vi "Parse Loaded Profile (uSMC).vi"(2 "replace(false)/insert(true)":bool, 3 "SMindex":i32, 4 "Version":string, 5 "data string":string) -> ()   [LabVIEW 2010, in "SignalWriterMH110203USBStepperMotor.lvclass"]
uses:
  SignalWriterMH110203USBStepperMotor.lvclass
  Get State Control (uSMC).ctl
  Set Parameters (uSMC).ctl
  class_data.vi
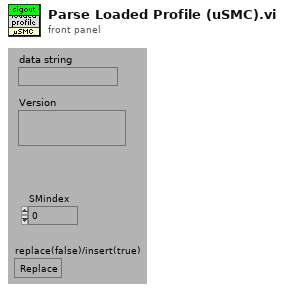
[diagram p1: front panel]
types:
  T1 = typedef "SignalWriterMH110203USBStepperMotor.lvclass/Get State Control (uSMC).ctl" = cluster{"Current Posistion":dbl, "CW/CCW":bool, "Speed":u16, "Temperature":dbl, "Power":u16, "Limit Switch 1":bool, "Limit Switch 2":bool, "After Reset":bool, "Step":u8, "Backlash":bool, "RT Error":bool, "RT State":bool, "Sync In":bool, "Sync Out":bool, "Ext Disconnect":bool, "Usb Powered":bool, "Voltage":dbl, "Working":bool, "SM Position in Encoder Units":i32, "Encoder Current Position":i32}
  T2 = typedef "SignalWriterMH110203USBStepperMotor.lvclass/Set Parameters (uSMC).ctl" = cluster{"Acceleration Time":u8, "Deceleration Time":u8, "Reduce Current Timeout":u16, "Buttons Timeout 1":u16, "Buttons Timeout 2":u16, "Buttons Timeout 3":u16, "Buttons Timeout 4":u16, "Buttons Timeout Reset":u16, "Buttons Timeout DblClick":u16, "Reset Speed":u16, "Buttons Speed 1":u16, "Buttons Speed 2":u16, "Buttons Speed 3":u16, "Buttons Speed 4":u16, "Max Backlash":u16, "Start Pos":i32, "RTdelta":u16, "RTMinError":u16, "Maximum Temperature":u16, "Sync Duration":u8, "Backlash Speed":u16, "EncVSCP":u8, "Steps Per Revolution":i32, "Encoder Pulses Per Rev-on":i32}
  T3 = cluster{"Cur Pos Units":dbl, "Set Cur Pos units":dbl, "Lo Limit Units":dbl, "Hi Limit Units":dbl, "Cur Pos Ticks":i32, "Set Cur Pos ticks":i32, "Lo Limit Ticks":i32, "Hi Limit Ticks":i32, "Minimal Value":dbl, "Maximal Value":dbl}
  T4 = typedef "SignalWriterMH110203USBStepperMotor.lvclass/Mode Control (uSMC).ctl" = cluster{"Turn Buttons Off":bool, "Reduce Current":bool, "Power Off and Make a Whole Step":bool, "Emergency Power Off":bool, "Limit Switch 1 True State":bool, "Limit Switch 2 True State":bool, "Rotary Transducer TRUE State":bool, "Swap Limit Switches":bool, "Limit Switch 1 Operation Enabled":bool, "Limit Switch 2 Operation Enabled":bool, "Rotary Transducer Operation Enabled":bool, "Rotary Transducer Operation Select":bool, "Button 1 True State":bool, "Button 2 True State":bool, "Swap Buttons":bool, "Reset Rotary Transducer Check Positions":bool, "Output Syncronization Enabled":bool, "Reset Output Sync Count":bool, "Sync Operation":bool, "Sync Count":u32, "Power":bool, "Invert Sync Polarity":bool, "Use Encoder":bool, "Invert Encoder Direction":bool, "Reset Encoder To 0":bool, "Reset SM Enc Pos to Enc Pos":bool}
  T5 = typedef "SignalWriterMH110203USBStepperMotor.lvclass/GoTo Control (uSMC).ctl" = cluster{"Step motor ID":string, "SMname":string, "Backlash":u16, "wait for input sygnal to start":bool, "use slow start/stop":bool, "units name":string, "Maximum speed":dbl, "speed":dbl, "step":u8, "point 1 ticks":i32, "point 2 ticks":i32, "point 1 units":dbl, "point 2 units":dbl, "Limit Switch standoff":dbl, "Zero Value":dbl, "Destination Position":dbl, "force backlash":bool, "power off when stop":bool, "POff delay":dbl, "positioner name":string, "R, Ohm":dbl, "I, mA":dbl, "Positioner's Type":u16, "Reset Direction":bool, "Manufacturer":string, "Model":string, "Scheme":string, "FirmwareVer":string}
  T6 = cluster{"Step motor ID":string, "SMname":string, "Loft":u16, "wait for input sygnal to start":bool, "use slow start/stop":bool, "units name":string, "Maximum speed":dbl, "speed":dbl, "step":u8, "point 1 ticks":i32, "point 2 ticks":i32, "point 1 units":dbl, "point 2 units":dbl, "Trailer 1 standoff":dbl, "Zero Value":dbl, "Destination Position":dbl, "force loft":bool, "power off when stop":bool, "POff delay":dbl, "positioner name":string, "R, Ohm":dbl, "I, mA":dbl, "Positioner's Type":u16, "Reset Direction":bool, "Manufacturer":string, "Model":string, "Scheme":string}
  T7 = cluster{"cur pos units":dbl, "set cur pos units value":dbl, "lo limit units":dbl, "hi limit units":dbl, "cur pos ticks":i32, "set cur pos ticks value":i32, "lo limit ticks":i32, "hi limit ticks":i32, "Minimal Value":dbl, "Maximal Value":dbl}
  T8 = cluster{"Step motor ID":string, "SMname":string, "Loft":u16, "wait for input sygnal to start":bool, "use slow start/stop":bool, "units name":string, "Maximum speed":dbl, "speed":dbl, "step":u8, "point 1 ticks":i32, "point 2 ticks":i32, "point 1 units":dbl, "point 2 units":dbl, "Trailer 1 standoff":dbl, "Zero Value":dbl, "Destination Position":dbl, "force loft":bool, "power off when stop":bool, "POff delay":dbl, "positioner name":string, "R, Ohm":dbl, "I, mA":dbl, "Positioner's Type":u16, "Reset Direction":bool, "Manufacturer":string, "Model":string, "Scheme":string, "FirmwareVer":string}
  T9 = cluster{"Turn Buttons Off":bool, "Reduce Current":bool, "Power Off and Make a Whole Step":bool, "Emergency Power Off":bool, "Trailer 1 True State":bool, "Trailer 2 True State":bool, "Rotary Transducer TRUE State":bool, "Swap Trailers":bool, "Trailer 1 Operation Enabled":bool, "Trailer 2 Operation Enabled":bool, "Rotary Transducer Operation Enabled":bool, "Rotary Transducer Operation Select":bool, "Button 1 True State":bool, "Button 2 True State":bool, "Swap Buttons":bool, "Reset Rotary Transducer Check Positions":bool, "Output Syncronization Enabled":bool, "Reset Output Sync Count":bool, "Sync Operation":bool, "Sync Count":u32, "Power":bool, "Invert Sync Polarity":bool, "Use Encoder":bool, "Invert Encoder Direction":bool, "Reset Encoder To 0":bool, "Reset SM Enc Pos to Enc Pos":bool}
  T10 = cluster{"Step motor ID":string, "SMname":string, "Loft":u16, "wait for input sygnal to start":bool, "use slow start/stop":bool, "units name":string, "Maximum speed":dbl, "speed":dbl, "step":u8, "point 1 ticks":i32, "point 2 ticks":i32, "point 1 units":dbl, "point 2 units":dbl, "Trailer 1 standoff":dbl, "Trailer 2 standoff":dbl, "Destination Position":dbl, "force loft":bool, "power off when stop":bool, "POff delay":dbl}
  T11 = cluster{"cur pos units":dbl, "set cur pos units value":dbl, "lo limit units":dbl, "hi limit units":dbl, "cur pos ticks":i32, "set cur pos ticks value":i32, "lo limit ticks":i32, "hi limit ticks":i32}
  T12 = cluster{"Delay 1":u8, "Delay 2":u8, "RefINTimeout":u16, "BTIMEOUT 1":u16, "BTIMEOUT 2":u16, "BTIMEOUT 3":u16, "BTIMEOUT 4":u16, "BTIMEOUT R":u16, "BTIMEOUT D":u16, "Min period":u16, "BTO1P":u16, "BTO2P":u16, "BTO3P":u16, "BTO4P":u16, "Max Loft":u16, "Start Pos":i32, "RTDelta":u16, "RTMinError":u16, "Maximum temperature":u16, "sync duration":u8, "LoftPeriod":u16}
  T13 = cluster{"buttons off":bool, "RefIin current":bool, "power off and make a whole step":bool, "emergency power off":bool, "trailer 1 true state":bool, "trailer 2 true state":bool, "Rotary Transducer TRUE state":bool, "trailers swap":bool, "trailer 1 operation enabled":bool, "trailer 2 operation enabled":bool, "Rotary Transducer Operation enabled":bool, "Rotary Transducer Operation select":bool, "Button 1 TRUE state":bool, "Button 2 TRUE state":bool, "Buttons are Swapped":bool, "Reset Rotary Transducer Check Positions":bool, "Output Syncronization Enabled":bool, "reset output sync count":bool, "Sync operation true-one time, false - many times":bool, "Sync count":u32, "power state":bool}
  T14 = cluster{"SetMode defalults":cluster{"buttons off":bool, "RefIin current":bool, "power off and make a whole step":bool, "emergency power off":bool, "trailer 1 true state":bool, "trailer 2 true state":bool, "Rotary Transducer TRUE state":bool, "trailers swap":bool, "trailer 1 operation enabled":bool, "trailer 2 operation enabled":bool, "Rotary Transducer Operation enabled":bool, "Rotary Transducer Operation select":bool, "Button 1 TRUE state":bool, "Button 2 TRUE state":bool, "Buttons are Swapped":bool, "Reset Rotary Transducer Check Positions":bool, "Output Syncronization Enabled":bool, "reset output sync count":bool, "Sync operation true-one time, false - many times":bool, "Sync count":u32, "power state":bool}, "SetParams Defalut":cluster{"Delay 1":u8, "Delay 2":u8, "RefINTimeout":u16, "BTIMEOUT 1":u16, "BTIMEOUT 2":u16, "BTIMEOUT 3":u16, "BTIMEOUT 4":u16, "BTIMEOUT R":u16, "BTIMEOUT D":u16, "Min period":u16, "BTO1P":u16, "BTO2P":u16, "BTO3P":u16, "BTO4P":u16, "Max Loft":u16, "Start Pos":i32, "RTDelta":u16, "RTMinError":u16, "Maximum temperature":u16, "sync duration":u8, "LoftPeriod":u16}, "Position Default":cluster{"cur pos units":dbl, "set cur pos units value":dbl, "lo limit units":dbl, "hi limit units":dbl, "cur pos ticks":i32, "set cur pos ticks value":i32, "lo limit ticks":i32, "hi limit ticks":i32}, "GoToPlus default":cluster{"Step motor ID":string, "SMname":string, "Loft":u16, "wait for input sygnal to start":bool, "use slow start/stop":bool, "units name":string, "Maximum speed":dbl, "speed":dbl, "step":u8, "point 1 ticks":i32, "point 2 ticks":i32, "point 1 units":dbl, "point 2 units":dbl, "Trailer 1 standoff":dbl, "Trailer 2 standoff":dbl, "Destination Position":dbl, "force loft":bool, "power off when stop":bool, "POff delay":dbl}}
  T15 = cluster{"Step motor ID":string, "SMname":string, "Loft":u16, "wait for input sygnal to start":bool, "use slow start/stop":bool, "units name":string, "Maximum speed":dbl, "speed":dbl, "step":u8, "point 1 ticks":i32, "point 2 ticks":i32, "point 1 units":dbl, "point 2 units":dbl, "Trailer 1 standoff":dbl, "Trailer 2 standoff":dbl, "Destination Position":dbl, "force loft":bool, "power off when stop":bool, "POff delay":dbl, "positioner name":string}
  T16 = cluster{"SetMode defalults":cluster{"buttons off":bool, "RefIin current":bool, "power off and make a whole step":bool, "emergency power off":bool, "trailer 1 true state":bool, "trailer 2 true state":bool, "Rotary Transducer TRUE state":bool, "trailers swap":bool, "trailer 1 operation enabled":bool, "trailer 2 operation enabled":bool, "Rotary Transducer Operation enabled":bool, "Rotary Transducer Operation select":bool, "Button 1 TRUE state":bool, "Button 2 TRUE state":bool, "Buttons are Swapped":bool, "Reset Rotary Transducer Check Positions":bool, "Output Syncronization Enabled":bool, "reset output sync count":bool, "Sync operation true-one time, false - many times":bool, "Sync count":u32, "power state":bool}, "SetParams Defalut":cluster{"Delay 1":u8, "Delay 2":u8, "RefINTimeout":u16, "BTIMEOUT 1":u16, "BTIMEOUT 2":u16, "BTIMEOUT 3":u16, "BTIMEOUT 4":u16, "BTIMEOUT R":u16, "BTIMEOUT D":u16, "Min period":u16, "BTO1P":u16, "BTO2P":u16, "BTO3P":u16, "BTO4P":u16, "Max Loft":u16, "Start Pos":i32, "RTDelta":u16, "RTMinError":u16, "Maximum temperature":u16, "sync duration":u8, "LoftPeriod":u16}, "Position Default":cluster{"cur pos units":dbl, "set cur pos units value":dbl, "lo limit units":dbl, "hi limit units":dbl, "cur pos ticks":i32, "set cur pos ticks value":i32, "lo limit ticks":i32, "hi limit ticks":i32}, "GoToPlus default":cluster{"Step motor ID":string, "SMname":string, "Loft":u16, "wait for input sygnal to start":bool, "use slow start/stop":bool, "units name":string, "Maximum speed":dbl, "speed":dbl, "step":u8, "point 1 ticks":i32, "point 2 ticks":i32, "point 1 units":dbl, "point 2 units":dbl, "Trailer 1 standoff":dbl, "Trailer 2 standoff":dbl, "Destination Position":dbl, "force loft":bool, "power off when stop":bool, "POff delay":dbl, "positioner name":string}}
  T17 = cluster{"SetMode defalults":cluster{"buttons off":bool, "RefIin current":bool, "power off and make a whole step":bool, "emergency power off":bool, "trailer 1 true state":bool, "trailer 2 true state":bool, "Rotary Transducer TRUE state":bool, "trailers swap":bool, "trailer 1 operation enabled":bool, "trailer 2 operation enabled":bool, "Rotary Transducer Operation enabled":bool, "Rotary Transducer Operation select":bool, "Button 1 TRUE state":bool, "Button 2 TRUE state":bool, "Buttons are Swapped":bool, "Reset Rotary Transducer Check Positions":bool, "Output Syncronization Enabled":bool, "reset output sync count":bool, "Sync operation true-one time, false - many times":bool, "Sync count":u32, "power state":bool}, "SetParams Defalut":cluster{"Delay 1":u8, "Delay 2":u8, "RefINTimeout":u16, "BTIMEOUT 1":u16, "BTIMEOUT 2":u16, "BTIMEOUT 3":u16, "BTIMEOUT 4":u16, "BTIMEOUT R":u16, "BTIMEOUT D":u16, "Min period":u16, "BTO1P":u16, "BTO2P":u16, "BTO3P":u16, "BTO4P":u16, "Max Loft":u16, "Start Pos":i32, "RTDelta":u16, "RTMinError":u16, "Maximum temperature":u16, "sync duration":u8, "LoftPeriod":u16}, "Position Default":cluster{"cur pos units":dbl, "set cur pos units value":dbl, "lo limit units":dbl, "hi limit units":dbl, "cur pos ticks":i32, "set cur pos ticks value":i32, "lo limit ticks":i32, "hi limit ticks":i32, "Minimal Value":dbl, "Maximal Value":dbl}, "GoToPlus default":cluster{"Step motor ID":string, "SMname":string, "Loft":u16, "wait for input sygnal to start":bool, "use slow start/stop":bool, "units name":string, "Maximum speed":dbl, "speed":dbl, "step":u8, "point 1 ticks":i32, "point 2 ticks":i32, "point 1 units":dbl, "point 2 units":dbl, "Trailer 1 standoff":dbl, "Zero Value":dbl, "Destination Position":dbl, "force loft":bool, "power off when stop":bool, "POff delay":dbl, "positioner name":string, "R, Ohm":dbl, "I, mA":dbl, "Positioner's Type":u16, "Reset Direction":bool, "Manufacturer":string, "Model":string, "Scheme":string}}
  T18 = cluster{"SetMode defalults":cluster{"buttons off":bool, "RefIin current":bool, "power off and make a whole step":bool, "emergency power off":bool, "trailer 1 true state":bool, "trailer 2 true state":bool, "Rotary Transducer TRUE state":bool, "trailers swap":bool, "trailer 1 operation enabled":bool, "trailer 2 operation enabled":bool, "Rotary Transducer Operation enabled":bool, "Rotary Transducer Operation select":bool, "Button 1 TRUE state":bool, "Button 2 TRUE state":bool, "Buttons are Swapped":bool, "Reset Rotary Transducer Check Positions":bool, "Output Syncronization Enabled":bool, "reset output sync count":bool, "Sync operation true-one time, false - many times":bool, "Sync count":u32, "power state":bool}, "SetParams Defalut":cluster{"Delay 1":u8, "Delay 2":u8, "RefINTimeout":u16, "BTIMEOUT 1":u16, "BTIMEOUT 2":u16, "BTIMEOUT 3":u16, "BTIMEOUT 4":u16, "BTIMEOUT R":u16, "BTIMEOUT D":u16, "Min period":u16, "BTO1P":u16, "BTO2P":u16, "BTO3P":u16, "BTO4P":u16, "Max Loft":u16, "Start Pos":i32, "RTDelta":u16, "RTMinError":u16, "Maximum temperature":u16, "sync duration":u8, "LoftPeriod":u16}, "Position Default":cluster{"cur pos units":dbl, "set cur pos units value":dbl, "lo limit units":dbl, "hi limit units":dbl, "cur pos ticks":i32, "set cur pos ticks value":i32, "lo limit ticks":i32, "hi limit ticks":i32, "Minimal Value":dbl, "Maximal Value":dbl}, "GoToPlus default":cluster{"Step motor ID":string, "SMname":string, "Loft":u16, "wait for input sygnal to start":bool, "use slow start/stop":bool, "units name":string, "Maximum speed":dbl, "speed":dbl, "step":u8, "point 1 ticks":i32, "point 2 ticks":i32, "point 1 units":dbl, "point 2 units":dbl, "Trailer 1 standoff":dbl, "Zero Value":dbl, "Destination Position":dbl, "force loft":bool, "power off when stop":bool, "POff delay":dbl, "positioner name":string, "R, Ohm":dbl, "I, mA":dbl, "Positioner's Type":u16, "Reset Direction":bool, "Manufacturer":string, "Model":string, "Scheme":string, "FirmwareVer":string}}
  T19 = cluster{"buttons off":bool, "RefIin current":bool, "power off and make a whole step":bool, "emergency power off":bool, "trailer 1 true state":bool, "trailer 2 true state":bool, "Rotary Transducer TRUE state":bool, "trailers swap":bool, "trailer 1 operation enabled":bool, "trailer 2 operation enabled":bool, "Rotary Transducer Operation enabled":bool, "Rotary Transducer Operation select":bool, "Button 1 TRUE state":bool, "Button 2 TRUE state":bool, "Buttons are Swapped":bool, "Reset Rotary Transducer Check Positions":bool, "Output Syncronization Enabled":bool, "reset output sync count":bool, "Sync operation true-one time, false - many times":bool, "Sync count":u32, "power state":bool, "Const TTL output":bool}
  T20 = cluster{"SetMode defalults":cluster{"buttons off":bool, "RefIin current":bool, "power off and make a whole step":bool, "emergency power off":bool, "trailer 1 true state":bool, "trailer 2 true state":bool, "Rotary Transducer TRUE state":bool, "trailers swap":bool, "trailer 1 operation enabled":bool, "trailer 2 operation enabled":bool, "Rotary Transducer Operation enabled":bool, "Rotary Transducer Operation select":bool, "Button 1 TRUE state":bool, "Button 2 TRUE state":bool, "Buttons are Swapped":bool, "Reset Rotary Transducer Check Positions":bool, "Output Syncronization Enabled":bool, "reset output sync count":bool, "Sync operation true-one time, false - many times":bool, "Sync count":u32, "power state":bool, "Const TTL output":bool}, "SetParams Defalut":cluster{"Delay 1":u8, "Delay 2":u8, "RefINTimeout":u16, "BTIMEOUT 1":u16, "BTIMEOUT 2":u16, "BTIMEOUT 3":u16, "BTIMEOUT 4":u16, "BTIMEOUT R":u16, "BTIMEOUT D":u16, "Min period":u16, "BTO1P":u16, "BTO2P":u16, "BTO3P":u16, "BTO4P":u16, "Max Loft":u16, "Start Pos":i32, "RTDelta":u16, "RTMinError":u16, "Maximum temperature":u16, "sync duration":u8, "LoftPeriod":u16}, "Position Default":cluster{"cur pos units":dbl, "set cur pos units value":dbl, "lo limit units":dbl, "hi limit units":dbl, "cur pos ticks":i32, "set cur pos ticks value":i32, "lo limit ticks":i32, "hi limit ticks":i32, "Minimal Value":dbl, "Maximal Value":dbl}, "GoToPlus default":cluster{"Step motor ID":string, "SMname":string, "Loft":u16, "wait for input sygnal to start":bool, "use slow start/stop":bool, "units name":string, "Maximum speed":dbl, "speed":dbl, "step":u8, "point 1 ticks":i32, "point 2 ticks":i32, "point 1 units":dbl, "point 2 units":dbl, "Trailer 1 standoff":dbl, "Zero Value":dbl, "Destination Position":dbl, "force loft":bool, "power off when stop":bool, "POff delay":dbl, "positioner name":string, "R, Ohm":dbl, "I, mA":dbl, "Positioner's Type":u16, "Reset Direction":bool, "Manufacturer":string, "Model":string, "Scheme":string, "FirmwareVer":string}}
  T21 = cluster{"Mode Defalults":cluster{"Turn Buttons Off":bool, "Reduce Current":bool, "Power Off and Make a Whole Step":bool, "Emergency Power Off":bool, "Trailer 1 True State":bool, "Trailer 2 True State":bool, "Rotary Transducer TRUE State":bool, "Swap Trailers":bool, "Trailer 1 Operation Enabled":bool, "Trailer 2 Operation Enabled":bool, "Rotary Transducer Operation Enabled":bool, "Rotary Transducer Operation Select":bool, "Button 1 True State":bool, "Button 2 True State":bool, "Swap Buttons":bool, "Reset Rotary Transducer Check Positions":bool, "Output Syncronization Enabled":bool, "Reset Output Sync Count":bool, "Sync Operation":bool, "Sync Count":u32, "Power":bool, "Invert Sync Polarity":bool, "Use Encoder":bool, "Invert Encoder Direction":bool, "Reset Encoder To 0":bool, "Reset SM Enc Pos to Enc Pos":bool}, "Parameters Defalut":T2, "Position Default":cluster{"cur pos units":dbl, "set cur pos units value":dbl, "lo limit units":dbl, "hi limit units":dbl, "cur pos ticks":i32, "set cur pos ticks value":i32, "lo limit ticks":i32, "hi limit ticks":i32, "Minimal Value":dbl, "Maximal Value":dbl}, "GoToPlus default":cluster{"Step motor ID":string, "SMname":string, "Loft":u16, "wait for input sygnal to start":bool, "use slow start/stop":bool, "units name":string, "Maximum speed":dbl, "speed":dbl, "step":u8, "point 1 ticks":i32, "point 2 ticks":i32, "point 1 units":dbl, "point 2 units":dbl, "Trailer 1 standoff":dbl, "Zero Value":dbl, "Destination Position":dbl, "force loft":bool, "power off when stop":bool, "POff delay":dbl, "positioner name":string, "R, Ohm":dbl, "I, mA":dbl, "Positioner's Type":u16, "Reset Direction":bool, "Manufacturer":string, "Model":string, "Scheme":string, "FirmwareVer":string}}
  T22 = cluster{"Mode Defalults":T4, "Parameters Defalut":T2, "Position Default":cluster{"Cur Pos Units":dbl, "Set Cur Pos units":dbl, "Lo Limit Units":dbl, "Hi Limit Units":dbl, "Cur Pos Ticks":i32, "Set Cur Pos ticks":i32, "Lo Limit Ticks":i32, "Hi Limit Ticks":i32, "Minimal Value":dbl, "Maximal Value":dbl}, "StartPlus Default":T5}
  T23 = cluster{"Cur Pos Units":dbl, "Set Cur Pos units":dbl, "Lo Limit Units":dbl, "Hi Limit Units":dbl, "Cur Pos Ticks":i32, "Set Cur Pos ticks":i32, "Lo Limit Ticks":i32, "Hi Limit Ticks":i32, "Minimal Value":dbl, "Maximal Value":dbl}[]
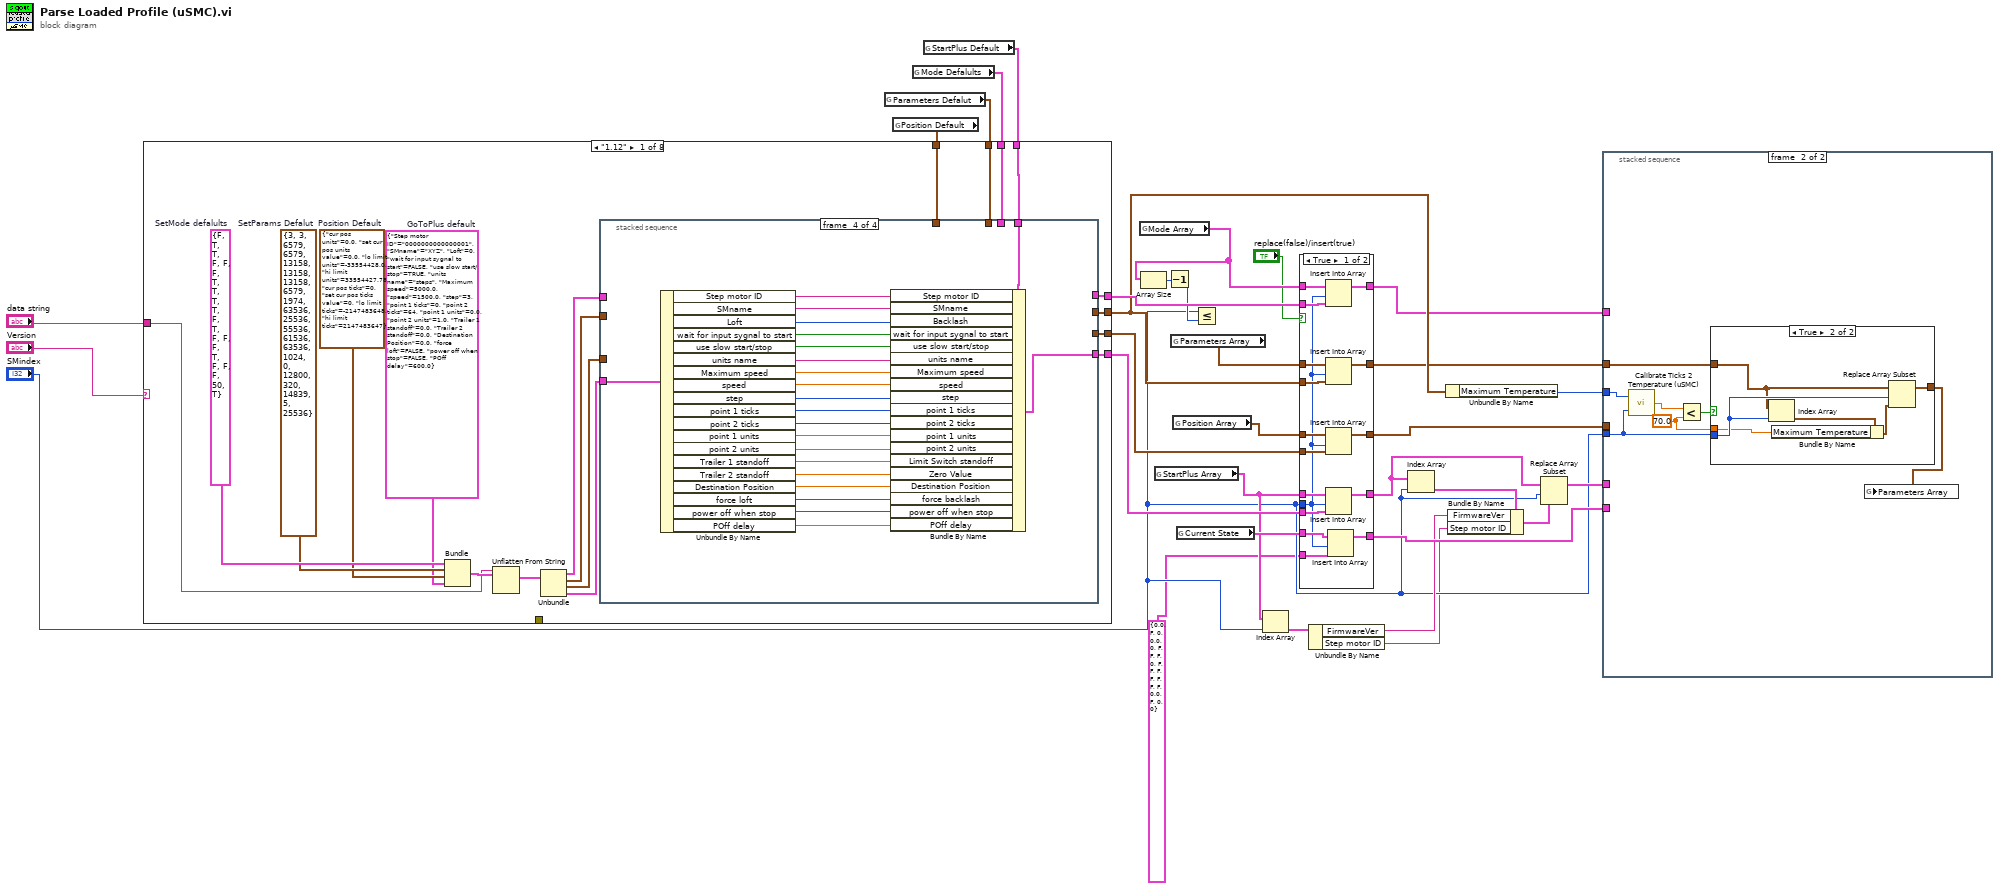
[diagram p0: block diagram]
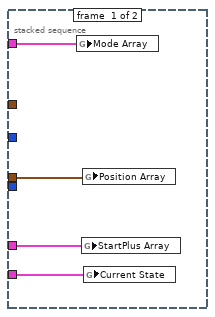
[diagram p2: hidden frame]
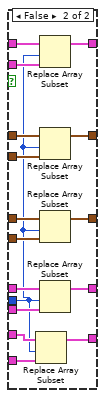
[diagram p4: hidden frame]
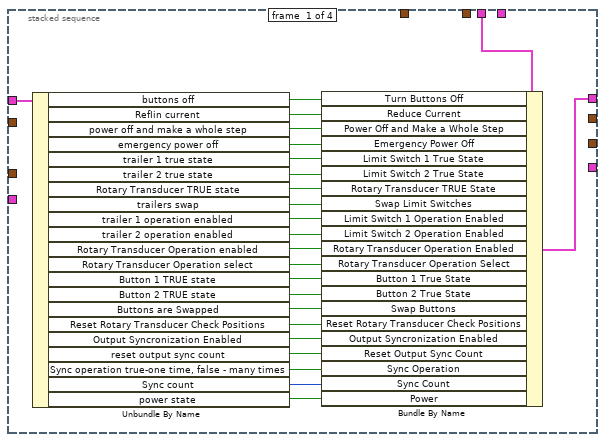
[diagram p5: hidden frame]
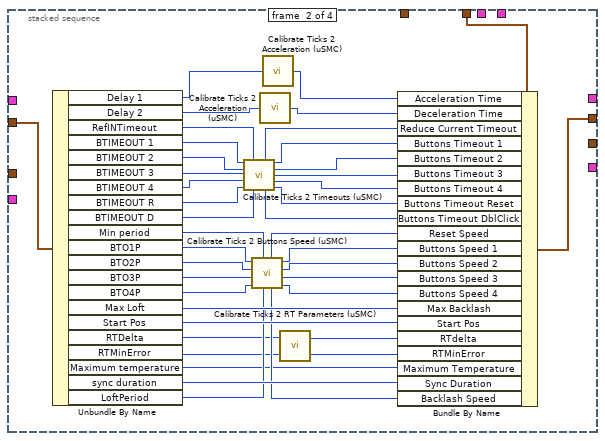
[diagram p6: hidden frame]
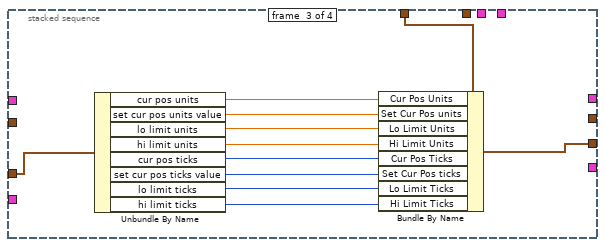
[diagram p7: hidden frame]
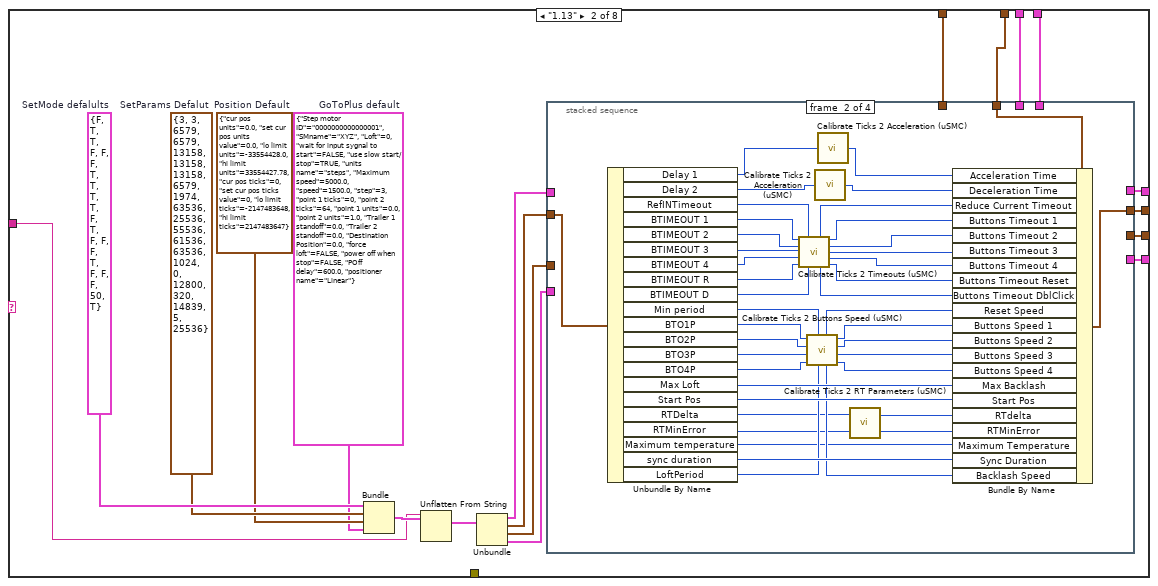
[diagram p8: hidden frame]
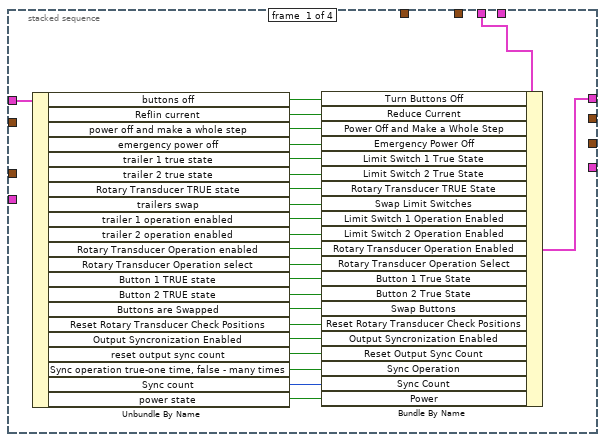
[diagram p9: hidden frame]
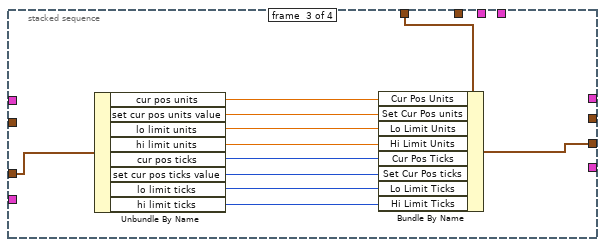
[diagram p10: hidden frame]
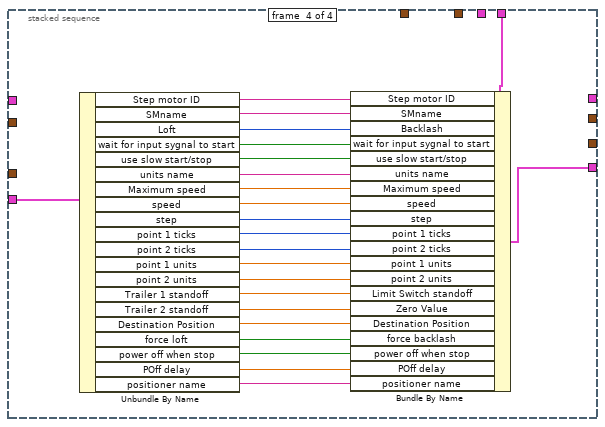
[diagram p11: hidden frame]
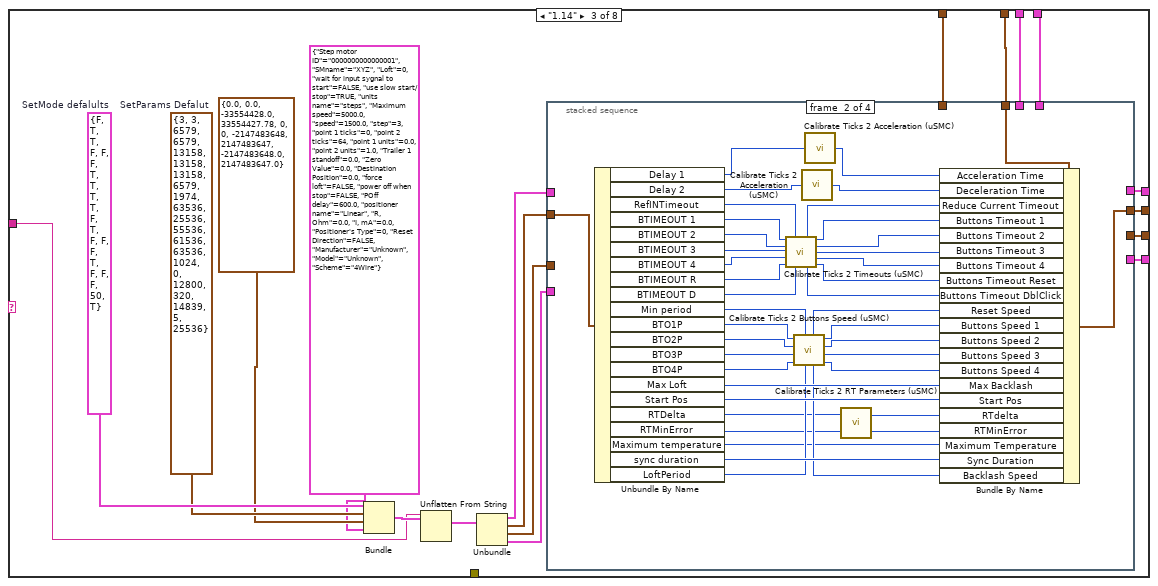
[diagram p12: hidden frame]
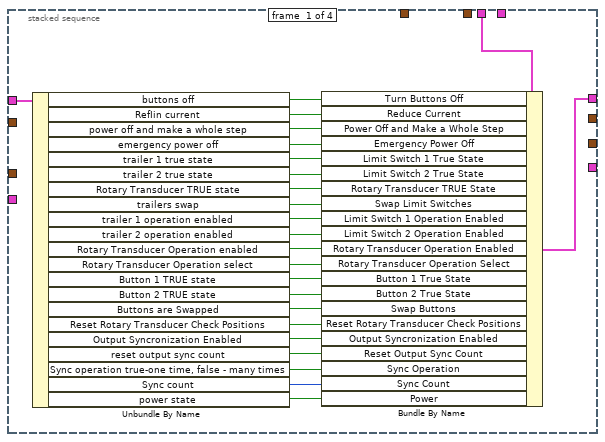
[diagram p13: hidden frame]
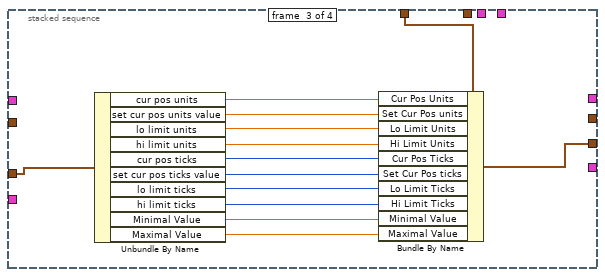
[diagram p14: hidden frame]
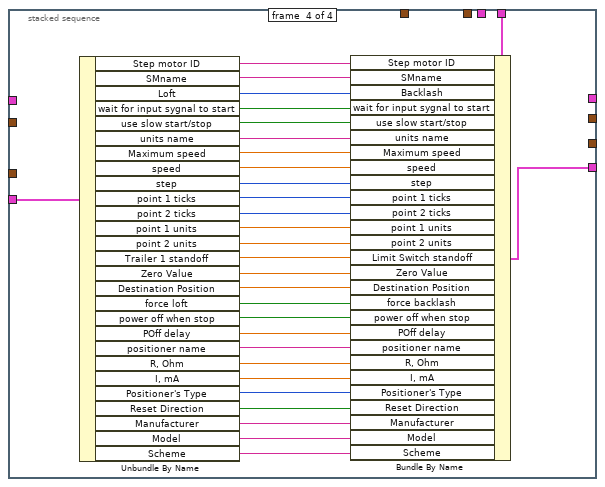
[diagram p15: hidden frame]
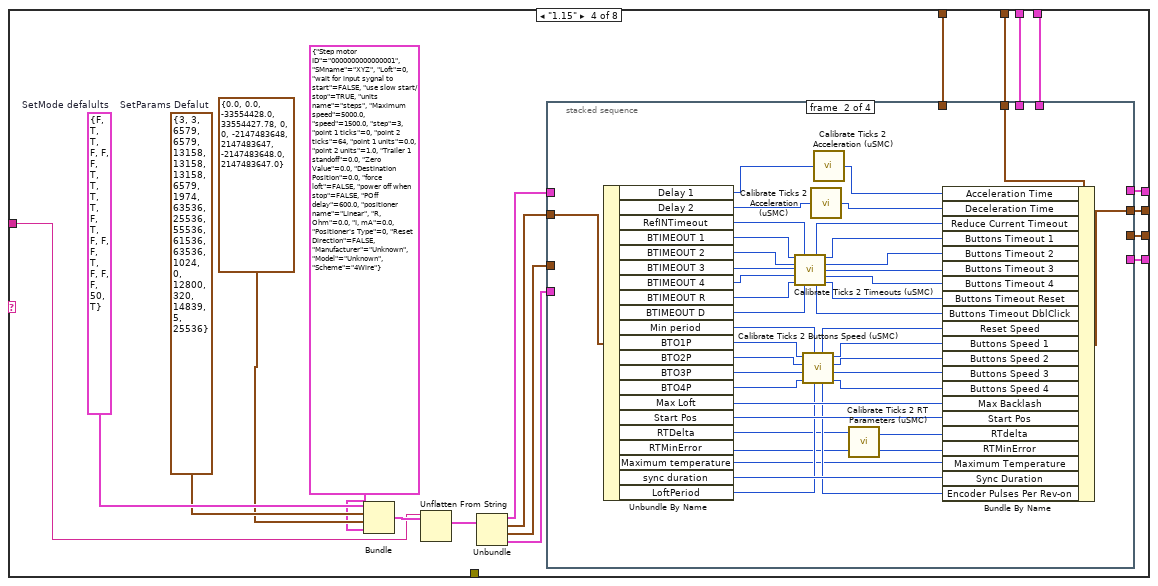
[diagram p16: hidden frame]
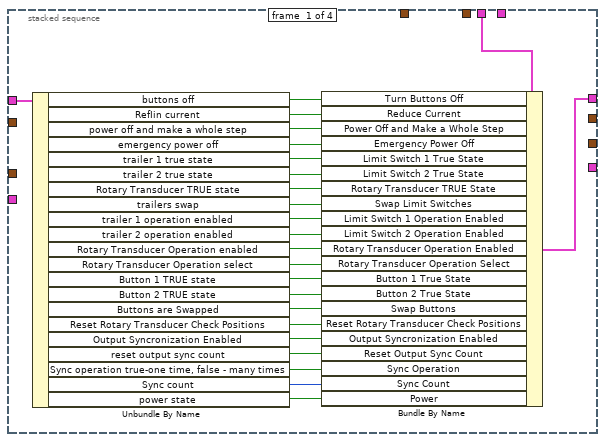
[diagram p17: hidden frame]
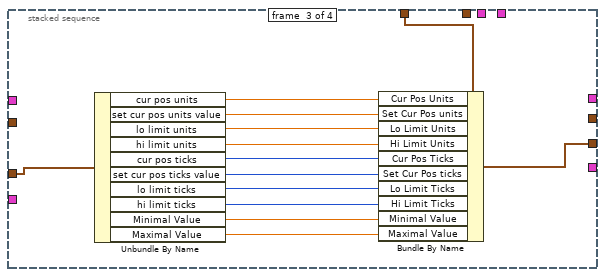
[diagram p18: hidden frame]
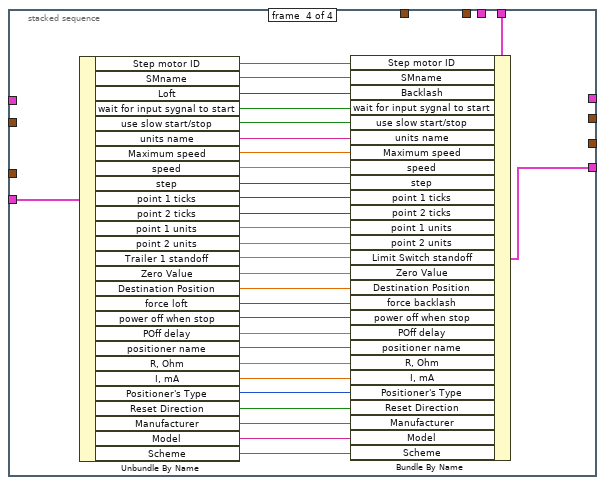
[diagram p19: hidden frame]
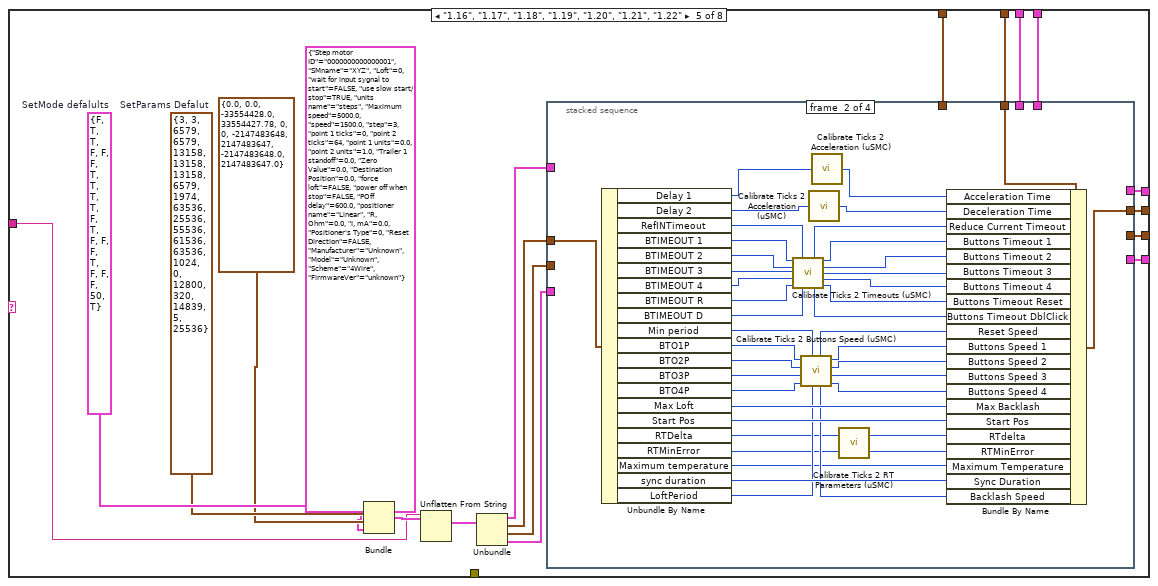
[diagram p20: hidden frame]
diagram:
  n1 = global read "class_data.vi" "Parameters Defalut"() -> (w1:T2)
  n2 = global read "class_data.vi" "Position Default"() -> (w2:T3)
  n3 = global read "class_data.vi" "Mode Defalults"() -> (w3:T4)
  n4 = global read "class_data.vi" "StartPlus Default"() -> (w4:T5)
  n5 = case shown="\"1.12\"" "Version" {
    tunnel: "data string" -> [w47 w163 w283 w410 w537 w664 w795 w924]
    tunnel: [w44 w160 w280 w407 w534 w661 w792 w922] -> w29
    tunnel: [w40 w157 w277 w404 w531 w657 w788 w920] -> w28
    tunnel: [w38 w155 w275 w402 w529 w655 w786 w919] -> w27
    tunnel: [w43 w150 w268 w395 w522 w660 w791 w921] -> w17
    tunnel: w4 -> [w36 w154 w270 w399 w526 w652 w783 w914]
    tunnel: w3 -> [w35 w153 w269 w398 w525 w651 w782 w917]
    tunnel: w1 -> [w34 w152 w272 w397 w524 w650 w781 w916]
    tunnel: w2 -> [w33 w151 w271 w396 w523 w649 w780 w915]
    tunnel: [_ _ _ _ _ _ w777 _] -> _
    frame "1.12" {
      w37 = T10 {"Step motor ID"="0000000000000001", "SMname"="XYZ", "Loft"=0, "wait for input sygnal to start"=FALSE, "use slow start/stop"=TRUE, "units name"="steps", "Maximum speed"=5000.0, "speed"=1500.0, "step"=3, "point 1 ticks"=0, "point 2 ticks"=64, "point 1 units"=0.0, "point 2 units"=1.0, "Trailer 1 standoff"=0.0, "Trailer 2 standoff"=0.0, "Destination Position"=0.0, "force loft"=FALSE, "power off when stop"=FALSE, "POff delay"=600.0}  # GoToPlus default
      w49 = T11 {"cur pos units"=0.0, "set cur pos units value"=0.0, "lo limit units"=-33554428.0, "hi limit units"=33554427.78, "cur pos ticks"=0, "set cur pos ticks value"=0, "lo limit ticks"=-2147483648, "hi limit ticks"=2147483647}  # Position Default
      w50 = T12 {"Delay 1"=3, "Delay 2"=3, "RefINTimeout"=6579, "BTIMEOUT 1"=6579, "BTIMEOUT 2"=13158, "BTIMEOUT 3"=13158, "BTIMEOUT 4"=13158, "BTIMEOUT R"=6579, "BTIMEOUT D"=1974, "Min period"=63536, "BTO1P"=25536, "BTO2P"=55536, "BTO3P"=61536, "BTO4P"=63536, "Max Loft"=1024, "Start Pos"=0, "RTDelta"=12800, "RTMinError"=320, "Maximum temperature"=14839, "sync duration"=5, "LoftPeriod"=25536}  # SetParams Defalut
      w51 = T13 {"buttons off"=FALSE, "RefIin current"=TRUE, "power off and make a whole step"=TRUE, "emergency power off"=FALSE, "trailer 1 true state"=FALSE, "trailer 2 true state"=FALSE, "Rotary Transducer TRUE state"=TRUE, "trailers swap"=TRUE, "trailer 1 operation enabled"=TRUE, "trailer 2 operation enabled"=TRUE, "Rotary Transducer Operation enabled"=FALSE, "Rotary Transducer Operation select"=TRUE, "Button 1 TRUE state"=FALSE, "Button 2 TRUE state"=FALSE, "Buttons are Swapped"=FALSE, "Reset Rotary Transducer Check Positions"=TRUE, "Output Syncronization Enabled"=FALSE, "reset output sync count"=FALSE, "Sync operation true-one time, false - many times"=FALSE, "Sync count"=50, "power state"=TRUE}  # SetMode defalults
      n6 = Bundle("SetMode defalults"=w51, "SetParams Defalut"=w50, "Position Default"=w49, "GoToPlus default"=w37) -> (w48:T14)  [unwired: 1 in]
      n7 = Unflatten From String(type=w48, binary string=w47) -> (value=w46:T14)  [unwired: 3 in, 2 out]
      n8 = Unbundle(w46) -> ("SetMode defalults"=w45:T13, "SetParams Defalut"=w42:T12, "Position Default"=w41:T11, "GoToPlus default"=w39:T10)
      n9 = stacked-sequence {
        tunnel: w45 -> [w75 _ _ _]
        tunnel: [w53 _ _ _] -> w44
        tunnel: [_ w80 _ _] -> w43
        tunnel: w42 -> [_ w82 _ _]
        tunnel: w41 -> [_ _ w119 _]
        tunnel: [_ _ w118 _] -> w40
        tunnel: w39 -> [_ _ _ w149]
        tunnel: [_ _ _ w130] -> w38
        tunnel: w36 -> [_ _ _ w128]
        tunnel: w35 -> [w52 _ _ _]
        tunnel: w34 -> [_ w81 _ _]
        tunnel: w33 -> [_ _ w117 _]
        frame #0 {
          n10 = Unbundle By Name(w75) -> ("buttons off"=w74:bool, "RefIin current"=w73:bool, "power off and make a whole step"=w72:bool, "emergency power off"=w71:bool, "trailer 1 true state"=w70:bool, "trailer 2 true state"=w69:bool, "Rotary Transducer TRUE state"=w68:bool, "trailers swap"=w67:bool, "trailer 1 operation enabled"=w66:bool, "trailer 2 operation enabled"=w65:bool, "Rotary Transducer Operation enabled"=w64:bool, "Rotary Transducer Operation select"=w63:bool, "Button 1 TRUE state"=w62:bool, "Button 2 TRUE state"=w61:bool, "Buttons are Swapped"=w60:bool, "Reset Rotary Transducer Check Positions"=w59:bool, "Output Syncronization Enabled"=w58:bool, "reset output sync count"=w56:bool, "Sync operation true-one time, false - many times"=w57:bool, "Sync count"=w55:u32, "power state"=w54:bool)
          n11 = Bundle By Name(cluster=w52, "Turn Buttons Off"=w74, "Reduce Current"=w73, "Power Off and Make a Whole Step"=w72, "Emergency Power Off"=w71, "Limit Switch 1 True State"=w70, "Limit Switch 2 True State"=w69, "Rotary Transducer TRUE State"=w68, "Swap Limit Switches"=w67, "Limit Switch 1 Operation Enabled"=w66, "Limit Switch 2 Operation Enabled"=w65, "Rotary Transducer Operation Enabled"=w64, "Rotary Transducer Operation Select"=w63, "Button 1 True State"=w62, "Button 2 True State"=w61, "Swap Buttons"=w60, "Reset Rotary Transducer Check Positions"=w59, "Output Syncronization Enabled"=w58, "Reset Output Sync Count"=w56, "Sync Operation"=w57, "Sync Count"=w55, "Power"=w54) -> (w53:T4)
        }
        frame #1 {
          n12 = Unbundle By Name(w82) -> ("Delay 1"=w84:u8, "Delay 2"=w86:u8, "RefINTimeout"=w113:u16, "BTIMEOUT 1"=w112:u16, "BTIMEOUT 2"=w111:u16, "BTIMEOUT 3"=w110:u16, "BTIMEOUT 4"=w109:u16, "BTIMEOUT R"=w108:u16, "BTIMEOUT D"=w107:u16, "Min period"=w99:u16, "BTO1P"=w98:u16, "BTO2P"=w97:u16, "BTO3P"=w96:u16, "BTO4P"=w95:u16, "Max Loft"=w116:u16, "Start Pos"=w115:i32, "RTDelta"=w79:u16, "RTMinError"=w78:u16, "Maximum temperature"=w87:u16, "sync duration"=w114:u8, "LoftPeriod"=w94:u16)
          n13 = call "Calibrate Ticks 2 Timeouts (uSMC).vi"("Buttons Timeout 1 (ticks)"=w112, "Reduce Current Timeout (ticks)"=w113, "Buttons Timeout 2 (ticks)"=w111, "Buttons Timeout 3 (ticks)"=w110, "Buttons Timeout 4 (ticks)"=w109, "Buttons Timeout Reset (ticks)"=w108, "Buttons Timeout DblClick (ticks)"=w107) -> ("Reduce Current Timeout (ms)"=w106:u16, "Buttons Timeout 1 (ms)"=w105:u16, "Buttons Timeout 2 (ms)"=w104:u16, "Buttons Timeout 3 (ms)"=w103:u16, "Buttons Timeout 4 (ms)"=w102:u16, "Buttons Timeout DblClick (ms)"=w100:u16, "Buttons Timeout Reset (ms)"=w101:u16)  [unwired: 2 in]
          n14 = call "Calibrate Ticks 2 Buttons Speed (uSMC).vi"("Backlash Speed (ticks)"=w94, "Reset Speed (ticks)"=w99, "Buttons Speed 4 (ticks)"=w95, "Buttons Speed 3 (ticks)"=w96, "Buttons Speed 2 (ticks)"=w97, "Buttons Speed 1 (ticks)"=w98) -> ("Buttons Speed 4 (Full Steps/Sec)"=w92:u16, "Buttons Speed 3 (Full Steps/Sec)"=w91:u16, "Buttons Speed 2 (Full Steps/Sec)"=w90:u16, "Buttons Speed 1 (Full Steps/Sec)"=w89:u16, "Backlash Speed (Full Steps/Sec)"=w93:u16, "Reset Speed (Full Steps/Sec)"=w88:u16)
          n15 = call "Calibrate Ticks 2 Acceleration (uSMC).vi"("Acceleration (ticks)"=w86) -> ("Acceleration (ms)"=w85:u16)
          n16 = call "Calibrate Ticks 2 Acceleration (uSMC).vi"("Acceleration (ticks)"=w84) -> ("Acceleration (ms)"=w83:u16)
          n17 = call "Calibrate Ticks 2 RT Parameters (uSMC).vi"("RTMinError (ticks)"=w78, "RTDelta (ticks)"=w79) -> ("RTMinError (a.u.)"=w76:u16, "RTDelta (a.u.)"=w77:u16)
          n18 = Bundle By Name(cluster=w81, "Acceleration Time"=w83, "Deceleration Time"=w85, "Reduce Current Timeout"=w106, "Buttons Timeout 1"=w105, "Buttons Timeout 2"=w104, "Buttons Timeout 3"=w103, "Buttons Timeout 4"=w102, "Buttons Timeout Reset"=w101, "Buttons Timeout DblClick"=w100, "Reset Speed"=w88, "Buttons Speed 1"=w89, "Buttons Speed 2"=w90, "Buttons Speed 3"=w91, "Buttons Speed 4"=w92, "Max Backlash"=w116, "Start Pos"=w115, "RTdelta"=w77, "RTMinError"=w76, "Maximum Temperature"=w87, "Sync Duration"=w114, "Backlash Speed"=w93) -> (w80:T2)
        }
        frame #2 {
          n19 = Unbundle By Name(w119) -> ("cur pos units"=w127:dbl, "set cur pos units value"=w126:dbl, "lo limit units"=w125:dbl, "hi limit units"=w124:dbl, "cur pos ticks"=w123:i32, "set cur pos ticks value"=w122:i32, "lo limit ticks"=w121:i32, "hi limit ticks"=w120:i32)
          n20 = Bundle By Name(cluster=w117, "Cur Pos Units"=w127, "Set Cur Pos units"=w126, "Lo Limit Units"=w125, "Hi Limit Units"=w124, "Cur Pos Ticks"=w123, "Set Cur Pos ticks"=w122, "Lo Limit Ticks"=w121, "Hi Limit Ticks"=w120) -> (w118:T3)
        }
        frame #3 {
          n21 = Unbundle By Name(w149) -> ("Step motor ID"=w129:string, "SMname"=w148:string, "Loft"=w147:u16, "wait for input sygnal to start"=w146:bool, "use slow start/stop"=w145:bool, "units name"=w144:string, "Maximum speed"=w143:dbl, "speed"=w142:dbl, "step"=w141:u8, "point 1 ticks"=w140:i32, "point 2 ticks"=w139:i32, "point 1 units"=w138:dbl, "point 2 units"=w137:dbl, "Trailer 1 standoff"=w136:dbl, "Trailer 2 standoff"=w135:dbl, "Destination Position"=w134:dbl, "force loft"=w133:bool, "power off when stop"=w132:bool, "POff delay"=w131:dbl)
          n22 = Bundle By Name(cluster=w128, "Step motor ID"=w129, "SMname"=w148, "Backlash"=w147, "wait for input sygnal to start"=w146, "use slow start/stop"=w145, "units name"=w144, "Maximum speed"=w143, "speed"=w142, "step"=w141, "point 1 ticks"=w140, "point 2 ticks"=w139, "point 1 units"=w138, "point 2 units"=w137, "Limit Switch standoff"=w136, "Zero Value"=w135, "Destination Position"=w134, "force backlash"=w133, "power off when stop"=w132, "POff delay"=w131) -> (w130:T5)
        }
      }
    }
    frame "1.13" {
      w165 = T15 {"Step motor ID"="0000000000000001", "SMname"="XYZ", "Loft"=0, "wait for input sygnal to start"=FALSE, "use slow start/stop"=TRUE, "units name"="steps", "Maximum speed"=5000.0, "speed"=1500.0, "step"=3, "point 1 ticks"=0, "point 2 ticks"=64, "point 1 units"=0.0, "point 2 units"=1.0, "Trailer 1 standoff"=0.0, "Trailer 2 standoff"=0.0, "Destination Position"=0.0, "force loft"=FALSE, "power off when stop"=FALSE, "POff delay"=600.0, "positioner name"="Linear"}  # GoToPlus default
      w166 = T11 {"cur pos units"=0.0, "set cur pos units value"=0.0, "lo limit units"=-33554428.0, "hi limit units"=33554427.78, "cur pos ticks"=0, "set cur pos ticks value"=0, "lo limit ticks"=-2147483648, "hi limit ticks"=2147483647}  # Position Default
      w167 = T12 {"Delay 1"=3, "Delay 2"=3, "RefINTimeout"=6579, "BTIMEOUT 1"=6579, "BTIMEOUT 2"=13158, "BTIMEOUT 3"=13158, "BTIMEOUT 4"=13158, "BTIMEOUT R"=6579, "BTIMEOUT D"=1974, "Min period"=63536, "BTO1P"=25536, "BTO2P"=55536, "BTO3P"=61536, "BTO4P"=63536, "Max Loft"=1024, "Start Pos"=0, "RTDelta"=12800, "RTMinError"=320, "Maximum temperature"=14839, "sync duration"=5, "LoftPeriod"=25536}  # SetParams Defalut
      w168 = T13 {"buttons off"=FALSE, "RefIin current"=TRUE, "power off and make a whole step"=TRUE, "emergency power off"=FALSE, "trailer 1 true state"=FALSE, "trailer 2 true state"=FALSE, "Rotary Transducer TRUE state"=TRUE, "trailers swap"=TRUE, "trailer 1 operation enabled"=TRUE, "trailer 2 operation enabled"=TRUE, "Rotary Transducer Operation enabled"=FALSE, "Rotary Transducer Operation select"=TRUE, "Button 1 TRUE state"=FALSE, "Button 2 TRUE state"=FALSE, "Buttons are Swapped"=FALSE, "Reset Rotary Transducer Check Positions"=TRUE, "Output Syncronization Enabled"=FALSE, "reset output sync count"=FALSE, "Sync operation true-one time, false - many times"=FALSE, "Sync count"=50, "power state"=TRUE}  # SetMode defalults
      n23 = Bundle("SetMode defalults"=w168, "SetParams Defalut"=w167, "Position Default"=w166, "GoToPlus default"=w165) -> (w164:T16)  [unwired: 1 in]
      n24 = Unflatten From String(type=w164, binary string=w163) -> (value=w162:T16)  [unwired: 3 in, 2 out]
      n25 = Unbundle(w162) -> ("SetMode defalults"=w161:T13, "SetParams Defalut"=w159:T12, "Position Default"=w158:T11, "GoToPlus default"=w156:T15)
      n26 = stacked-sequence {
        tunnel: w161 -> [w192 _ _ _]
        tunnel: [w170 _ _ _] -> w160
        tunnel: w159 -> [_ w199 _ _]
        tunnel: w158 -> [_ _ w236 _]
        tunnel: [_ _ w235 _] -> w157
        tunnel: w156 -> [_ _ _ w267]
        tunnel: [_ _ _ w247] -> w155
        tunnel: w154 -> [_ _ _ w245]
        tunnel: w153 -> [w169 _ _ _]
        tunnel: w152 -> [_ w198 _ _]
        tunnel: w151 -> [_ _ w234 _]
        tunnel: [_ w197 _ _] -> w150
        frame #0 {
          n27 = Unbundle By Name(w192) -> ("buttons off"=w191:bool, "RefIin current"=w190:bool, "power off and make a whole step"=w189:bool, "emergency power off"=w188:bool, "trailer 1 true state"=w187:bool, "trailer 2 true state"=w186:bool, "Rotary Transducer TRUE state"=w185:bool, "trailers swap"=w184:bool, "trailer 1 operation enabled"=w183:bool, "trailer 2 operation enabled"=w182:bool, "Rotary Transducer Operation enabled"=w181:bool, "Rotary Transducer Operation select"=w180:bool, "Button 1 TRUE state"=w179:bool, "Button 2 TRUE state"=w178:bool, "Buttons are Swapped"=w177:bool, "Reset Rotary Transducer Check Positions"=w176:bool, "Output Syncronization Enabled"=w175:bool, "reset output sync count"=w173:bool, "Sync operation true-one time, false - many times"=w174:bool, "Sync count"=w172:u32, "power state"=w171:bool)
          n28 = Bundle By Name(cluster=w169, "Turn Buttons Off"=w191, "Reduce Current"=w190, "Power Off and Make a Whole Step"=w189, "Emergency Power Off"=w188, "Limit Switch 1 True State"=w187, "Limit Switch 2 True State"=w186, "Rotary Transducer TRUE State"=w185, "Swap Limit Switches"=w184, "Limit Switch 1 Operation Enabled"=w183, "Limit Switch 2 Operation Enabled"=w182, "Rotary Transducer Operation Enabled"=w181, "Rotary Transducer Operation Select"=w180, "Button 1 True State"=w179, "Button 2 True State"=w178, "Swap Buttons"=w177, "Reset Rotary Transducer Check Positions"=w176, "Output Syncronization Enabled"=w175, "Reset Output Sync Count"=w173, "Sync Operation"=w174, "Sync Count"=w172, "Power"=w171) -> (w170:T4)
        }
        frame #1 {
          n29 = Unbundle By Name(w199) -> ("Delay 1"=w201:u8, "Delay 2"=w203:u8, "RefINTimeout"=w230:u16, "BTIMEOUT 1"=w229:u16, "BTIMEOUT 2"=w228:u16, "BTIMEOUT 3"=w227:u16, "BTIMEOUT 4"=w226:u16, "BTIMEOUT R"=w225:u16, "BTIMEOUT D"=w224:u16, "Min period"=w216:u16, "BTO1P"=w215:u16, "BTO2P"=w214:u16, "BTO3P"=w213:u16, "BTO4P"=w212:u16, "Max Loft"=w233:u16, "Start Pos"=w232:i32, "RTDelta"=w196:u16, "RTMinError"=w195:u16, "Maximum temperature"=w204:u16, "sync duration"=w231:u8, "LoftPeriod"=w211:u16)
          n30 = call "Calibrate Ticks 2 Timeouts (uSMC).vi"("Buttons Timeout 1 (ticks)"=w229, "Reduce Current Timeout (ticks)"=w230, "Buttons Timeout 2 (ticks)"=w228, "Buttons Timeout 3 (ticks)"=w227, "Buttons Timeout 4 (ticks)"=w226, "Buttons Timeout Reset (ticks)"=w225, "Buttons Timeout DblClick (ticks)"=w224) -> ("Reduce Current Timeout (ms)"=w223:u16, "Buttons Timeout 1 (ms)"=w222:u16, "Buttons Timeout 2 (ms)"=w221:u16, "Buttons Timeout 3 (ms)"=w220:u16, "Buttons Timeout 4 (ms)"=w219:u16, "Buttons Timeout DblClick (ms)"=w217:u16, "Buttons Timeout Reset (ms)"=w218:u16)  [unwired: 2 in]
          n31 = call "Calibrate Ticks 2 Buttons Speed (uSMC).vi"("Backlash Speed (ticks)"=w211, "Reset Speed (ticks)"=w216, "Buttons Speed 4 (ticks)"=w212, "Buttons Speed 3 (ticks)"=w213, "Buttons Speed 2 (ticks)"=w214, "Buttons Speed 1 (ticks)"=w215) -> ("Buttons Speed 4 (Full Steps/Sec)"=w209:u16, "Buttons Speed 3 (Full Steps/Sec)"=w208:u16, "Buttons Speed 2 (Full Steps/Sec)"=w207:u16, "Buttons Speed 1 (Full Steps/Sec)"=w206:u16, "Backlash Speed (Full Steps/Sec)"=w210:u16, "Reset Speed (Full Steps/Sec)"=w205:u16)
          n32 = call "Calibrate Ticks 2 Acceleration (uSMC).vi"("Acceleration (ticks)"=w203) -> ("Acceleration (ms)"=w202:u16)
          n33 = call "Calibrate Ticks 2 Acceleration (uSMC).vi"("Acceleration (ticks)"=w201) -> ("Acceleration (ms)"=w200:u16)
          n34 = call "Calibrate Ticks 2 RT Parameters (uSMC).vi"("RTMinError (ticks)"=w195, "RTDelta (ticks)"=w196) -> ("RTMinError (a.u.)"=w193:u16, "RTDelta (a.u.)"=w194:u16)
          n35 = Bundle By Name(cluster=w198, "Acceleration Time"=w200, "Deceleration Time"=w202, "Reduce Current Timeout"=w223, "Buttons Timeout 1"=w222, "Buttons Timeout 2"=w221, "Buttons Timeout 3"=w220, "Buttons Timeout 4"=w219, "Buttons Timeout Reset"=w218, "Buttons Timeout DblClick"=w217, "Reset Speed"=w205, "Buttons Speed 1"=w206, "Buttons Speed 2"=w207, "Buttons Speed 3"=w208, "Buttons Speed 4"=w209, "Max Backlash"=w233, "Start Pos"=w232, "RTdelta"=w194, "RTMinError"=w193, "Maximum Temperature"=w204, "Sync Duration"=w231, "Backlash Speed"=w210) -> (w197:T2)
        }
        frame #2 {
          n36 = Unbundle By Name(w236) -> ("cur pos units"=w244:dbl, "set cur pos units value"=w243:dbl, "lo limit units"=w242:dbl, "hi limit units"=w241:dbl, "cur pos ticks"=w240:i32, "set cur pos ticks value"=w239:i32, "lo limit ticks"=w238:i32, "hi limit ticks"=w237:i32)
          n37 = Bundle By Name(cluster=w234, "Cur Pos Units"=w244, "Set Cur Pos units"=w243, "Lo Limit Units"=w242, "Hi Limit Units"=w241, "Cur Pos Ticks"=w240, "Set Cur Pos ticks"=w239, "Lo Limit Ticks"=w238, "Hi Limit Ticks"=w237) -> (w235:T3)
        }
        frame #3 {
          n38 = Unbundle By Name(w267) -> ("Step motor ID"=w246:string, "SMname"=w266:string, "Loft"=w265:u16, "wait for input sygnal to start"=w264:bool, "use slow start/stop"=w263:bool, "units name"=w262:string, "Maximum speed"=w261:dbl, "speed"=w260:dbl, "step"=w259:u8, "point 1 ticks"=w258:i32, "point 2 ticks"=w257:i32, "point 1 units"=w256:dbl, "point 2 units"=w255:dbl, "Trailer 1 standoff"=w254:dbl, "Trailer 2 standoff"=w253:dbl, "Destination Position"=w252:dbl, "force loft"=w251:bool, "power off when stop"=w250:bool, "POff delay"=w249:dbl, "positioner name"=w248:string)
          n39 = Bundle By Name(cluster=w245, "Step motor ID"=w246, "SMname"=w266, "Backlash"=w265, "wait for input sygnal to start"=w264, "use slow start/stop"=w263, "units name"=w262, "Maximum speed"=w261, "speed"=w260, "step"=w259, "point 1 ticks"=w258, "point 2 ticks"=w257, "point 1 units"=w256, "point 2 units"=w255, "Limit Switch standoff"=w254, "Zero Value"=w253, "Destination Position"=w252, "force backlash"=w251, "power off when stop"=w250, "POff delay"=w249, "positioner name"=w248) -> (w247:T5)
        }
      }
    }
    frame "1.14" {
      w285 = T12 {"Delay 1"=3, "Delay 2"=3, "RefINTimeout"=6579, "BTIMEOUT 1"=6579, "BTIMEOUT 2"=13158, "BTIMEOUT 3"=13158, "BTIMEOUT 4"=13158, "BTIMEOUT R"=6579, "BTIMEOUT D"=1974, "Min period"=63536, "BTO1P"=25536, "BTO2P"=55536, "BTO3P"=61536, "BTO4P"=63536, "Max Loft"=1024, "Start Pos"=0, "RTDelta"=12800, "RTMinError"=320, "Maximum temperature"=14839, "sync duration"=5, "LoftPeriod"=25536}  # SetParams Defalut
      w286 = T13 {"buttons off"=FALSE, "RefIin current"=TRUE, "power off and make a whole step"=TRUE, "emergency power off"=FALSE, "trailer 1 true state"=FALSE, "trailer 2 true state"=FALSE, "Rotary Transducer TRUE state"=TRUE, "trailers swap"=TRUE, "trailer 1 operation enabled"=TRUE, "trailer 2 operation enabled"=TRUE, "Rotary Transducer Operation enabled"=FALSE, "Rotary Transducer Operation select"=TRUE, "Button 1 TRUE state"=FALSE, "Button 2 TRUE state"=FALSE, "Buttons are Swapped"=FALSE, "Reset Rotary Transducer Check Positions"=TRUE, "Output Syncronization Enabled"=FALSE, "reset output sync count"=FALSE, "Sync operation true-one time, false - many times"=FALSE, "Sync count"=50, "power state"=TRUE}  # SetMode defalults
      n40 = Bundle("SetMode defalults"=w286, "SetParams Defalut"=w285, "Position Default"=T7 {"cur pos units"=0.0, "set cur pos units value"=0.0, "lo limit units"=-33554428.0, "hi limit units"=33554427.78, "cur pos ticks"=0, "set cur pos ticks value"=0, "lo limit ticks"=-2147483648, "hi limit ticks"=2147483647, "Minimal Value"=-2147483648.0, "Maximal Value"=2147483647.0}, "GoToPlus default"=T6 {"Step motor ID"="0000000000000001", "SMname"="XYZ", "Loft"=0, "wait for input sygnal to start"=FALSE, "use slow start/stop"=TRUE, "units name"="steps", "Maximum speed"=5000.0, "speed"=1500.0, "step"=3, "point 1 ticks"=0, "point 2 ticks"=64, "point 1 units"=0.0, "point 2 units"=1.0, "Trailer 1 standoff"=0.0, "Zero Value"=0.0, "Destination Position"=0.0, "force loft"=FALSE, "power off when stop"=FALSE, "POff delay"=600.0, "positioner name"="Linear", "R, Ohm"=0.0, "I, mA"=0.0, "Positioner's Type"=0, "Reset Direction"=FALSE, "Manufacturer"="Unknown", "Model"="Unknown", "Scheme"="4Wire"}) -> (w284:T17)  [unwired: 1 in]
      n41 = Unflatten From String(type=w284, binary string=w283) -> (value=w282:T17)  [unwired: 3 in, 2 out]
      n42 = Unbundle(w282) -> ("SetMode defalults"=w281:T13, "SetParams Defalut"=w279:T12, "Position Default"=w278:T7, "GoToPlus default"=w276:T6)
      n43 = stacked-sequence {
        tunnel: w281 -> [w310 _ _ _]
        tunnel: [w288 _ _ _] -> w280
        tunnel: w279 -> [_ w315 _ _]
        tunnel: w278 -> [_ _ w356 _]
        tunnel: [_ _ w355 _] -> w277
        tunnel: w276 -> [_ _ _ w394]
        tunnel: [_ _ _ w374] -> w275
        tunnel: w272 -> [_ w317 _ _]
        tunnel: w271 -> [_ _ w352 _]
        tunnel: w270 -> [_ _ _ w365]
        tunnel: w269 -> [w287 _ _ _]
        tunnel: [_ w316 _ _] -> w268
        frame #0 {
          n44 = Unbundle By Name(w310) -> ("buttons off"=w309:bool, "RefIin current"=w308:bool, "power off and make a whole step"=w307:bool, "emergency power off"=w306:bool, "trailer 1 true state"=w305:bool, "trailer 2 true state"=w304:bool, "Rotary Transducer TRUE state"=w303:bool, "trailers swap"=w302:bool, "trailer 1 operation enabled"=w301:bool, "trailer 2 operation enabled"=w300:bool, "Rotary Transducer Operation enabled"=w299:bool, "Rotary Transducer Operation select"=w298:bool, "Button 1 TRUE state"=w297:bool, "Button 2 TRUE state"=w296:bool, "Buttons are Swapped"=w295:bool, "Reset Rotary Transducer Check Positions"=w294:bool, "Output Syncronization Enabled"=w293:bool, "reset output sync count"=w291:bool, "Sync operation true-one time, false - many times"=w292:bool, "Sync count"=w290:u32, "power state"=w289:bool)
          n45 = Bundle By Name(cluster=w287, "Turn Buttons Off"=w309, "Reduce Current"=w308, "Power Off and Make a Whole Step"=w307, "Emergency Power Off"=w306, "Limit Switch 1 True State"=w305, "Limit Switch 2 True State"=w304, "Rotary Transducer TRUE State"=w303, "Swap Limit Switches"=w302, "Limit Switch 1 Operation Enabled"=w301, "Limit Switch 2 Operation Enabled"=w300, "Rotary Transducer Operation Enabled"=w299, "Rotary Transducer Operation Select"=w298, "Button 1 True State"=w297, "Button 2 True State"=w296, "Swap Buttons"=w295, "Reset Rotary Transducer Check Positions"=w294, "Output Syncronization Enabled"=w293, "Reset Output Sync Count"=w291, "Sync Operation"=w292, "Sync Count"=w290, "Power"=w289) -> (w288:T4)
        }
        frame #1 {
          n46 = Unbundle By Name(w315) -> ("Delay 1"=w319:u8, "Delay 2"=w321:u8, "RefINTimeout"=w348:u16, "BTIMEOUT 1"=w347:u16, "BTIMEOUT 2"=w346:u16, "BTIMEOUT 3"=w345:u16, "BTIMEOUT 4"=w344:u16, "BTIMEOUT R"=w343:u16, "BTIMEOUT D"=w342:u16, "Min period"=w334:u16, "BTO1P"=w333:u16, "BTO2P"=w332:u16, "BTO3P"=w331:u16, "BTO4P"=w330:u16, "Max Loft"=w351:u16, "Start Pos"=w350:i32, "RTDelta"=w314:u16, "RTMinError"=w313:u16, "Maximum temperature"=w322:u16, "sync duration"=w349:u8, "LoftPeriod"=w329:u16)
          n47 = call "Calibrate Ticks 2 Timeouts (uSMC).vi"("Buttons Timeout 1 (ticks)"=w347, "Reduce Current Timeout (ticks)"=w348, "Buttons Timeout 2 (ticks)"=w346, "Buttons Timeout 3 (ticks)"=w345, "Buttons Timeout 4 (ticks)"=w344, "Buttons Timeout Reset (ticks)"=w343, "Buttons Timeout DblClick (ticks)"=w342) -> ("Reduce Current Timeout (ms)"=w341:u16, "Buttons Timeout 1 (ms)"=w340:u16, "Buttons Timeout 2 (ms)"=w339:u16, "Buttons Timeout 3 (ms)"=w338:u16, "Buttons Timeout 4 (ms)"=w337:u16, "Buttons Timeout DblClick (ms)"=w335:u16, "Buttons Timeout Reset (ms)"=w336:u16)  [unwired: 2 in]
          n48 = call "Calibrate Ticks 2 Buttons Speed (uSMC).vi"("Backlash Speed (ticks)"=w329, "Reset Speed (ticks)"=w334, "Buttons Speed 4 (ticks)"=w330, "Buttons Speed 3 (ticks)"=w331, "Buttons Speed 2 (ticks)"=w332, "Buttons Speed 1 (ticks)"=w333) -> ("Buttons Speed 4 (Full Steps/Sec)"=w327:u16, "Buttons Speed 3 (Full Steps/Sec)"=w326:u16, "Buttons Speed 2 (Full Steps/Sec)"=w325:u16, "Buttons Speed 1 (Full Steps/Sec)"=w324:u16, "Backlash Speed (Full Steps/Sec)"=w328:u16, "Reset Speed (Full Steps/Sec)"=w323:u16)
          n49 = call "Calibrate Ticks 2 Acceleration (uSMC).vi"("Acceleration (ticks)"=w321) -> ("Acceleration (ms)"=w320:u16)
          n50 = call "Calibrate Ticks 2 Acceleration (uSMC).vi"("Acceleration (ticks)"=w319) -> ("Acceleration (ms)"=w318:u16)
          n51 = call "Calibrate Ticks 2 RT Parameters (uSMC).vi"("RTMinError (ticks)"=w313, "RTDelta (ticks)"=w314) -> ("RTMinError (a.u.)"=w311:u16, "RTDelta (a.u.)"=w312:u16)
          n52 = Bundle By Name(cluster=w317, "Acceleration Time"=w318, "Deceleration Time"=w320, "Reduce Current Timeout"=w341, "Buttons Timeout 1"=w340, "Buttons Timeout 2"=w339, "Buttons Timeout 3"=w338, "Buttons Timeout 4"=w337, "Buttons Timeout Reset"=w336, "Buttons Timeout DblClick"=w335, "Reset Speed"=w323, "Buttons Speed 1"=w324, "Buttons Speed 2"=w325, "Buttons Speed 3"=w326, "Buttons Speed 4"=w327, "Max Backlash"=w351, "Start Pos"=w350, "RTdelta"=w312, "RTMinError"=w311, "Maximum Temperature"=w322, "Sync Duration"=w349, "Backlash Speed"=w328) -> (w316:T2)
        }
        frame #2 {
          n53 = Unbundle By Name(w356) -> ("cur pos units"=w364:dbl, "set cur pos units value"=w363:dbl, "lo limit units"=w362:dbl, "hi limit units"=w361:dbl, "cur pos ticks"=w360:i32, "set cur pos ticks value"=w359:i32, "lo limit ticks"=w358:i32, "hi limit ticks"=w357:i32, "Minimal Value"=w354:dbl, "Maximal Value"=w353:dbl)
          n54 = Bundle By Name(cluster=w352, "Cur Pos Units"=w364, "Set Cur Pos units"=w363, "Lo Limit Units"=w362, "Hi Limit Units"=w361, "Cur Pos Ticks"=w360, "Set Cur Pos ticks"=w359, "Lo Limit Ticks"=w358, "Hi Limit Ticks"=w357, "Minimal Value"=w354, "Maximal Value"=w353) -> (w355:T3)
        }
        frame #3 {
          n55 = Unbundle By Name(w394) -> ("Step motor ID"=w369:string, "SMname"=w393:string, "Loft"=w392:u16, "wait for input sygnal to start"=w391:bool, "use slow start/stop"=w390:bool, "units name"=w389:string, "Maximum speed"=w388:dbl, "speed"=w387:dbl, "step"=w386:u8, "point 1 ticks"=w385:i32, "point 2 ticks"=w384:i32, "point 1 units"=w383:dbl, "point 2 units"=w382:dbl, "Trailer 1 standoff"=w381:dbl, "Zero Value"=w380:dbl, "Destination Position"=w379:dbl, "force loft"=w378:bool, "power off when stop"=w377:bool, "POff delay"=w376:dbl, "positioner name"=w375:string, "R, Ohm"=w373:dbl, "I, mA"=w372:dbl, "Positioner's Type"=w371:u16, "Reset Direction"=w370:bool, "Manufacturer"=w368:string, "Model"=w367:string, "Scheme"=w366:string)
          n56 = Bundle By Name(cluster=w365, "Step motor ID"=w369, "SMname"=w393, "Backlash"=w392, "wait for input sygnal to start"=w391, "use slow start/stop"=w390, "units name"=w389, "Maximum speed"=w388, "speed"=w387, "step"=w386, "point 1 ticks"=w385, "point 2 ticks"=w384, "point 1 units"=w383, "point 2 units"=w382, "Limit Switch standoff"=w381, "Zero Value"=w380, "Destination Position"=w379, "force backlash"=w378, "power off when stop"=w377, "POff delay"=w376, "positioner name"=w375, "R, Ohm"=w373, "I, mA"=w372, "Positioner's Type"=w371, "Reset Direction"=w370, "Manufacturer"=w368, "Model"=w367, "Scheme"=w366) -> (w374:T5)
        }
      }
    }
    frame "1.15" {
      w412 = T12 {"Delay 1"=3, "Delay 2"=3, "RefINTimeout"=6579, "BTIMEOUT 1"=6579, "BTIMEOUT 2"=13158, "BTIMEOUT 3"=13158, "BTIMEOUT 4"=13158, "BTIMEOUT R"=6579, "BTIMEOUT D"=1974, "Min period"=63536, "BTO1P"=25536, "BTO2P"=55536, "BTO3P"=61536, "BTO4P"=63536, "Max Loft"=1024, "Start Pos"=0, "RTDelta"=12800, "RTMinError"=320, "Maximum temperature"=14839, "sync duration"=5, "LoftPeriod"=25536}  # SetParams Defalut
      w413 = T13 {"buttons off"=FALSE, "RefIin current"=TRUE, "power off and make a whole step"=TRUE, "emergency power off"=FALSE, "trailer 1 true state"=FALSE, "trailer 2 true state"=FALSE, "Rotary Transducer TRUE state"=TRUE, "trailers swap"=TRUE, "trailer 1 operation enabled"=TRUE, "trailer 2 operation enabled"=TRUE, "Rotary Transducer Operation enabled"=FALSE, "Rotary Transducer Operation select"=TRUE, "Button 1 TRUE state"=FALSE, "Button 2 TRUE state"=FALSE, "Buttons are Swapped"=FALSE, "Reset Rotary Transducer Check Positions"=TRUE, "Output Syncronization Enabled"=FALSE, "reset output sync count"=FALSE, "Sync operation true-one time, false - many times"=FALSE, "Sync count"=50, "power state"=TRUE}  # SetMode defalults
      n57 = Bundle("SetMode defalults"=w413, "SetParams Defalut"=w412, "Position Default"=T7 {"cur pos units"=0.0, "set cur pos units value"=0.0, "lo limit units"=-33554428.0, "hi limit units"=33554427.78, "cur pos ticks"=0, "set cur pos ticks value"=0, "lo limit ticks"=-2147483648, "hi limit ticks"=2147483647, "Minimal Value"=-2147483648.0, "Maximal Value"=2147483647.0}, "GoToPlus default"=T6 {"Step motor ID"="0000000000000001", "SMname"="XYZ", "Loft"=0, "wait for input sygnal to start"=FALSE, "use slow start/stop"=TRUE, "units name"="steps", "Maximum speed"=5000.0, "speed"=1500.0, "step"=3, "point 1 ticks"=0, "point 2 ticks"=64, "point 1 units"=0.0, "point 2 units"=1.0, "Trailer 1 standoff"=0.0, "Zero Value"=0.0, "Destination Position"=0.0, "force loft"=FALSE, "power off when stop"=FALSE, "POff delay"=600.0, "positioner name"="Linear", "R, Ohm"=0.0, "I, mA"=0.0, "Positioner's Type"=0, "Reset Direction"=FALSE, "Manufacturer"="Unknown", "Model"="Unknown", "Scheme"="4Wire"}) -> (w411:T17)  [unwired: 1 in]
      n58 = Unflatten From String(type=w411, binary string=w410) -> (value=w409:T17)  [unwired: 3 in, 2 out]
      n59 = Unbundle(w409) -> ("SetMode defalults"=w408:T13, "SetParams Defalut"=w406:T12, "Position Default"=w405:T7, "GoToPlus default"=w403:T6)
      n60 = stacked-sequence {
        tunnel: w408 -> [w437 _ _ _]
        tunnel: [w415 _ _ _] -> w407
        tunnel: w406 -> [_ w442 _ _]
        tunnel: w405 -> [_ _ w483 _]
        tunnel: [_ _ w482 _] -> w404
        tunnel: w403 -> [_ _ _ w521]
        tunnel: [_ _ _ w501] -> w402
        tunnel: w399 -> [_ _ _ w492]
        tunnel: w398 -> [w414 _ _ _]
        tunnel: w397 -> [_ w443 _ _]
        tunnel: w396 -> [_ _ w479 _]
        tunnel: [_ w444 _ _] -> w395
        frame #0 {
          n61 = Unbundle By Name(w437) -> ("buttons off"=w436:bool, "RefIin current"=w435:bool, "power off and make a whole step"=w434:bool, "emergency power off"=w433:bool, "trailer 1 true state"=w432:bool, "trailer 2 true state"=w431:bool, "Rotary Transducer TRUE state"=w430:bool, "trailers swap"=w429:bool, "trailer 1 operation enabled"=w428:bool, "trailer 2 operation enabled"=w427:bool, "Rotary Transducer Operation enabled"=w426:bool, "Rotary Transducer Operation select"=w425:bool, "Button 1 TRUE state"=w424:bool, "Button 2 TRUE state"=w423:bool, "Buttons are Swapped"=w422:bool, "Reset Rotary Transducer Check Positions"=w421:bool, "Output Syncronization Enabled"=w420:bool, "reset output sync count"=w418:bool, "Sync operation true-one time, false - many times"=w419:bool, "Sync count"=w417:u32, "power state"=w416:bool)
          n62 = Bundle By Name(cluster=w414, "Turn Buttons Off"=w436, "Reduce Current"=w435, "Power Off and Make a Whole Step"=w434, "Emergency Power Off"=w433, "Limit Switch 1 True State"=w432, "Limit Switch 2 True State"=w431, "Rotary Transducer TRUE State"=w430, "Swap Limit Switches"=w429, "Limit Switch 1 Operation Enabled"=w428, "Limit Switch 2 Operation Enabled"=w427, "Rotary Transducer Operation Enabled"=w426, "Rotary Transducer Operation Select"=w425, "Button 1 True State"=w424, "Button 2 True State"=w423, "Swap Buttons"=w422, "Reset Rotary Transducer Check Positions"=w421, "Output Syncronization Enabled"=w420, "Reset Output Sync Count"=w418, "Sync Operation"=w419, "Sync Count"=w417, "Power"=w416) -> (w415:T4)
        }
        frame #1 {
          n63 = Unbundle By Name(w442) -> ("Delay 1"=w446:u8, "Delay 2"=w448:u8, "RefINTimeout"=w475:u16, "BTIMEOUT 1"=w474:u16, "BTIMEOUT 2"=w473:u16, "BTIMEOUT 3"=w472:u16, "BTIMEOUT 4"=w471:u16, "BTIMEOUT R"=w470:u16, "BTIMEOUT D"=w469:u16, "Min period"=w461:u16, "BTO1P"=w460:u16, "BTO2P"=w459:u16, "BTO3P"=w458:u16, "BTO4P"=w457:u16, "Max Loft"=w478:u16, "Start Pos"=w477:i32, "RTDelta"=w441:u16, "RTMinError"=w440:u16, "Maximum temperature"=w449:u16, "sync duration"=w476:u8, "LoftPeriod"=w456:u16)
          n64 = call "Calibrate Ticks 2 Timeouts (uSMC).vi"("Buttons Timeout 1 (ticks)"=w474, "Reduce Current Timeout (ticks)"=w475, "Buttons Timeout 2 (ticks)"=w473, "Buttons Timeout 3 (ticks)"=w472, "Buttons Timeout 4 (ticks)"=w471, "Buttons Timeout Reset (ticks)"=w470, "Buttons Timeout DblClick (ticks)"=w469) -> ("Reduce Current Timeout (ms)"=w468:u16, "Buttons Timeout 1 (ms)"=w467:u16, "Buttons Timeout 2 (ms)"=w466:u16, "Buttons Timeout 3 (ms)"=w465:u16, "Buttons Timeout 4 (ms)"=w464:u16, "Buttons Timeout DblClick (ms)"=w462:u16, "Buttons Timeout Reset (ms)"=w463:u16)  [unwired: 2 in]
          n65 = call "Calibrate Ticks 2 Buttons Speed (uSMC).vi"("Backlash Speed (ticks)"=w456, "Reset Speed (ticks)"=w461, "Buttons Speed 4 (ticks)"=w457, "Buttons Speed 3 (ticks)"=w458, "Buttons Speed 2 (ticks)"=w459, "Buttons Speed 1 (ticks)"=w460) -> ("Buttons Speed 4 (Full Steps/Sec)"=w454:u16, "Buttons Speed 3 (Full Steps/Sec)"=w453:u16, "Buttons Speed 2 (Full Steps/Sec)"=w452:u16, "Buttons Speed 1 (Full Steps/Sec)"=w451:u16, "Backlash Speed (Full Steps/Sec)"=w455:u16, "Reset Speed (Full Steps/Sec)"=w450:u16)
          n66 = call "Calibrate Ticks 2 Acceleration (uSMC).vi"("Acceleration (ticks)"=w448) -> ("Acceleration (ms)"=w447:u16)
          n67 = call "Calibrate Ticks 2 Acceleration (uSMC).vi"("Acceleration (ticks)"=w446) -> ("Acceleration (ms)"=w445:u16)
          n68 = call "Calibrate Ticks 2 RT Parameters (uSMC).vi"("RTMinError (ticks)"=w440, "RTDelta (ticks)"=w441) -> ("RTMinError (a.u.)"=w438:u16, "RTDelta (a.u.)"=w439:u16)
          n69 = Bundle By Name(cluster=w443, "Acceleration Time"=w445, "Deceleration Time"=w447, "Reduce Current Timeout"=w468, "Buttons Timeout 1"=w467, "Buttons Timeout 2"=w466, "Buttons Timeout 3"=w465, "Buttons Timeout 4"=w464, "Buttons Timeout Reset"=w463, "Buttons Timeout DblClick"=w462, "Reset Speed"=w450, "Buttons Speed 1"=w451, "Buttons Speed 2"=w452, "Buttons Speed 3"=w453, "Buttons Speed 4"=w454, "Max Backlash"=w478, "Start Pos"=w477, "RTdelta"=w439, "RTMinError"=w438, "Maximum Temperature"=w449, "Sync Duration"=w476, "Encoder Pulses Per Rev-on"=w455) -> (w444:T2)
        }
        frame #2 {
          n70 = Unbundle By Name(w483) -> ("cur pos units"=w491:dbl, "set cur pos units value"=w490:dbl, "lo limit units"=w489:dbl, "hi limit units"=w488:dbl, "cur pos ticks"=w487:i32, "set cur pos ticks value"=w486:i32, "lo limit ticks"=w485:i32, "hi limit ticks"=w484:i32, "Minimal Value"=w481:dbl, "Maximal Value"=w480:dbl)
          n71 = Bundle By Name(cluster=w479, "Cur Pos Units"=w491, "Set Cur Pos units"=w490, "Lo Limit Units"=w489, "Hi Limit Units"=w488, "Cur Pos Ticks"=w487, "Set Cur Pos ticks"=w486, "Lo Limit Ticks"=w485, "Hi Limit Ticks"=w484, "Minimal Value"=w481, "Maximal Value"=w480) -> (w482:T3)
        }
        frame #3 {
          n72 = Unbundle By Name(w521) -> ("Step motor ID"=w496:string, "SMname"=w520:string, "Loft"=w519:u16, "wait for input sygnal to start"=w518:bool, "use slow start/stop"=w517:bool, "units name"=w516:string, "Maximum speed"=w515:dbl, "speed"=w514:dbl, "step"=w513:u8, "point 1 ticks"=w512:i32, "point 2 ticks"=w511:i32, "point 1 units"=w510:dbl, "point 2 units"=w509:dbl, "Trailer 1 standoff"=w508:dbl, "Zero Value"=w507:dbl, "Destination Position"=w506:dbl, "force loft"=w505:bool, "power off when stop"=w504:bool, "POff delay"=w503:dbl, "positioner name"=w502:string, "R, Ohm"=w500:dbl, "I, mA"=w499:dbl, "Positioner's Type"=w498:u16, "Reset Direction"=w497:bool, "Manufacturer"=w495:string, "Model"=w494:string, "Scheme"=w493:string)
          n73 = Bundle By Name(cluster=w492, "Step motor ID"=w496, "SMname"=w520, "Backlash"=w519, "wait for input sygnal to start"=w518, "use slow start/stop"=w517, "units name"=w516, "Maximum speed"=w515, "speed"=w514, "step"=w513, "point 1 ticks"=w512, "point 2 ticks"=w511, "point 1 units"=w510, "point 2 units"=w509, "Limit Switch standoff"=w508, "Zero Value"=w507, "Destination Position"=w506, "force backlash"=w505, "power off when stop"=w504, "POff delay"=w503, "positioner name"=w502, "R, Ohm"=w500, "I, mA"=w499, "Positioner's Type"=w498, "Reset Direction"=w497, "Manufacturer"=w495, "Model"=w494, "Scheme"=w493) -> (w501:T5)
        }
      }
    }
    frame "1.16", "1.17", "1.18", "1.19", "1.20", "1.21", "1.22" {
      w539 = T12 {"Delay 1"=3, "Delay 2"=3, "RefINTimeout"=6579, "BTIMEOUT 1"=6579, "BTIMEOUT 2"=13158, "BTIMEOUT 3"=13158, "BTIMEOUT 4"=13158, "BTIMEOUT R"=6579, "BTIMEOUT D"=1974, "Min period"=63536, "BTO1P"=25536, "BTO2P"=55536, "BTO3P"=61536, "BTO4P"=63536, "Max Loft"=1024, "Start Pos"=0, "RTDelta"=12800, "RTMinError"=320, "Maximum temperature"=14839, "sync duration"=5, "LoftPeriod"=25536}  # SetParams Defalut
      w540 = T13 {"buttons off"=FALSE, "RefIin current"=TRUE, "power off and make a whole step"=TRUE, "emergency power off"=FALSE, "trailer 1 true state"=FALSE, "trailer 2 true state"=FALSE, "Rotary Transducer TRUE state"=TRUE, "trailers swap"=TRUE, "trailer 1 operation enabled"=TRUE, "trailer 2 operation enabled"=TRUE, "Rotary Transducer Operation enabled"=FALSE, "Rotary Transducer Operation select"=TRUE, "Button 1 TRUE state"=FALSE, "Button 2 TRUE state"=FALSE, "Buttons are Swapped"=FALSE, "Reset Rotary Transducer Check Positions"=TRUE, "Output Syncronization Enabled"=FALSE, "reset output sync count"=FALSE, "Sync operation true-one time, false - many times"=FALSE, "Sync count"=50, "power state"=TRUE}  # SetMode defalults
      n74 = Bundle("SetMode defalults"=w540, "SetParams Defalut"=w539, "Position Default"=T7 {"cur pos units"=0.0, "set cur pos units value"=0.0, "lo limit units"=-33554428.0, "hi limit units"=33554427.78, "cur pos ticks"=0, "set cur pos ticks value"=0, "lo limit ticks"=-2147483648, "hi limit ticks"=2147483647, "Minimal Value"=-2147483648.0, "Maximal Value"=2147483647.0}, "GoToPlus default"=T8 {"Step motor ID"="0000000000000001", "SMname"="XYZ", "Loft"=0, "wait for input sygnal to start"=FALSE, "use slow start/stop"=TRUE, "units name"="steps", "Maximum speed"=5000.0, "speed"=1500.0, "step"=3, "point 1 ticks"=0, "point 2 ticks"=64, "point 1 units"=0.0, "point 2 units"=1.0, "Trailer 1 standoff"=0.0, "Zero Value"=0.0, "Destination Position"=0.0, "force loft"=FALSE, "power off when stop"=FALSE, "POff delay"=600.0, "positioner name"="Linear", "R, Ohm"=0.0, "I, mA"=0.0, "Positioner's Type"=0, "Reset Direction"=FALSE, "Manufacturer"="Unknown", "Model"="Unknown", "Scheme"="4Wire", "FirmwareVer"="unknown"}) -> (w538:T18)  [unwired: 1 in]
      n75 = Unflatten From String(type=w538, binary string=w537) -> (value=w536:T18)  [unwired: 3 in, 2 out]
      n76 = Unbundle(w536) -> ("SetMode defalults"=w535:T13, "SetParams Defalut"=w533:T12, "Position Default"=w532:T7, "GoToPlus default"=w530:T8)
      n77 = stacked-sequence {
        tunnel: w535 -> [w564 _ _ _]
        tunnel: [w542 _ _ _] -> w534
        tunnel: w533 -> [_ w569 _ _]
        tunnel: w532 -> [_ _ w610 _]
        tunnel: [_ _ w609 _] -> w531
        tunnel: w530 -> [_ _ _ w648]
        tunnel: [_ _ _ w628] -> w529
        tunnel: w526 -> [_ _ _ w619]
        tunnel: w525 -> [w541 _ _ _]
        tunnel: w524 -> [_ w570 _ _]
        tunnel: w523 -> [_ _ w606 _]
        tunnel: [_ w571 _ _] -> w522
        frame #0 {
          n78 = Unbundle By Name(w564) -> ("buttons off"=w563:bool, "RefIin current"=w562:bool, "power off and make a whole step"=w561:bool, "emergency power off"=w560:bool, "trailer 1 true state"=w559:bool, "trailer 2 true state"=w558:bool, "Rotary Transducer TRUE state"=w557:bool, "trailers swap"=w556:bool, "trailer 1 operation enabled"=w555:bool, "trailer 2 operation enabled"=w554:bool, "Rotary Transducer Operation enabled"=w553:bool, "Rotary Transducer Operation select"=w552:bool, "Button 1 TRUE state"=w551:bool, "Button 2 TRUE state"=w550:bool, "Buttons are Swapped"=w549:bool, "Reset Rotary Transducer Check Positions"=w548:bool, "Output Syncronization Enabled"=w547:bool, "reset output sync count"=w545:bool, "Sync operation true-one time, false - many times"=w546:bool, "Sync count"=w544:u32, "power state"=w543:bool)
          n79 = Bundle By Name(cluster=w541, "Turn Buttons Off"=w563, "Reduce Current"=w562, "Power Off and Make a Whole Step"=w561, "Emergency Power Off"=w560, "Limit Switch 1 True State"=w559, "Limit Switch 2 True State"=w558, "Rotary Transducer TRUE State"=w557, "Swap Limit Switches"=w556, "Limit Switch 1 Operation Enabled"=w555, "Limit Switch 2 Operation Enabled"=w554, "Rotary Transducer Operation Enabled"=w553, "Rotary Transducer Operation Select"=w552, "Button 1 True State"=w551, "Button 2 True State"=w550, "Swap Buttons"=w549, "Reset Rotary Transducer Check Positions"=w548, "Output Syncronization Enabled"=w547, "Reset Output Sync Count"=w545, "Sync Operation"=w546, "Sync Count"=w544, "Power"=w543) -> (w542:T4)
        }
        frame #1 {
          n80 = Unbundle By Name(w569) -> ("Delay 1"=w573:u8, "Delay 2"=w575:u8, "RefINTimeout"=w602:u16, "BTIMEOUT 1"=w601:u16, "BTIMEOUT 2"=w600:u16, "BTIMEOUT 3"=w599:u16, "BTIMEOUT 4"=w598:u16, "BTIMEOUT R"=w597:u16, "BTIMEOUT D"=w596:u16, "Min period"=w588:u16, "BTO1P"=w587:u16, "BTO2P"=w586:u16, "BTO3P"=w585:u16, "BTO4P"=w584:u16, "Max Loft"=w605:u16, "Start Pos"=w604:i32, "RTDelta"=w568:u16, "RTMinError"=w567:u16, "Maximum temperature"=w576:u16, "sync duration"=w603:u8, "LoftPeriod"=w583:u16)
          n81 = call "Calibrate Ticks 2 Timeouts (uSMC).vi"("Buttons Timeout 1 (ticks)"=w601, "Reduce Current Timeout (ticks)"=w602, "Buttons Timeout 2 (ticks)"=w600, "Buttons Timeout 3 (ticks)"=w599, "Buttons Timeout 4 (ticks)"=w598, "Buttons Timeout Reset (ticks)"=w597, "Buttons Timeout DblClick (ticks)"=w596) -> ("Reduce Current Timeout (ms)"=w595:u16, "Buttons Timeout 1 (ms)"=w594:u16, "Buttons Timeout 2 (ms)"=w593:u16, "Buttons Timeout 3 (ms)"=w592:u16, "Buttons Timeout 4 (ms)"=w591:u16, "Buttons Timeout DblClick (ms)"=w589:u16, "Buttons Timeout Reset (ms)"=w590:u16)  [unwired: 2 in]
          n82 = call "Calibrate Ticks 2 Buttons Speed (uSMC).vi"("Backlash Speed (ticks)"=w583, "Reset Speed (ticks)"=w588, "Buttons Speed 4 (ticks)"=w584, "Buttons Speed 3 (ticks)"=w585, "Buttons Speed 2 (ticks)"=w586, "Buttons Speed 1 (ticks)"=w587) -> ("Buttons Speed 4 (Full Steps/Sec)"=w581:u16, "Buttons Speed 3 (Full Steps/Sec)"=w580:u16, "Buttons Speed 2 (Full Steps/Sec)"=w579:u16, "Buttons Speed 1 (Full Steps/Sec)"=w578:u16, "Backlash Speed (Full Steps/Sec)"=w582:u16, "Reset Speed (Full Steps/Sec)"=w577:u16)
          n83 = call "Calibrate Ticks 2 Acceleration (uSMC).vi"("Acceleration (ticks)"=w575) -> ("Acceleration (ms)"=w574:u16)
          n84 = call "Calibrate Ticks 2 Acceleration (uSMC).vi"("Acceleration (ticks)"=w573) -> ("Acceleration (ms)"=w572:u16)
          n85 = call "Calibrate Ticks 2 RT Parameters (uSMC).vi"("RTMinError (ticks)"=w567, "RTDelta (ticks)"=w568) -> ("RTMinError (a.u.)"=w565:u16, "RTDelta (a.u.)"=w566:u16)
          n86 = Bundle By Name(cluster=w570, "Acceleration Time"=w572, "Deceleration Time"=w574, "Reduce Current Timeout"=w595, "Buttons Timeout 1"=w594, "Buttons Timeout 2"=w593, "Buttons Timeout 3"=w592, "Buttons Timeout 4"=w591, "Buttons Timeout Reset"=w590, "Buttons Timeout DblClick"=w589, "Reset Speed"=w577, "Buttons Speed 1"=w578, "Buttons Speed 2"=w579, "Buttons Speed 3"=w580, "Buttons Speed 4"=w581, "Max Backlash"=w605, "Start Pos"=w604, "RTdelta"=w566, "RTMinError"=w565, "Maximum Temperature"=w576, "Sync Duration"=w603, "Backlash Speed"=w582) -> (w571:T2)
        }
        frame #2 {
          n87 = Unbundle By Name(w610) -> ("cur pos units"=w618:dbl, "set cur pos units value"=w617:dbl, "lo limit units"=w616:dbl, "hi limit units"=w615:dbl, "cur pos ticks"=w614:i32, "set cur pos ticks value"=w613:i32, "lo limit ticks"=w612:i32, "hi limit ticks"=w611:i32, "Minimal Value"=w608:dbl, "Maximal Value"=w607:dbl)
          n88 = Bundle By Name(cluster=w606, "Cur Pos Units"=w618, "Set Cur Pos units"=w617, "Lo Limit Units"=w616, "Hi Limit Units"=w615, "Cur Pos Ticks"=w614, "Set Cur Pos ticks"=w613, "Lo Limit Ticks"=w612, "Hi Limit Ticks"=w611, "Minimal Value"=w608, "Maximal Value"=w607) -> (w609:T3)
        }
        frame #3 {
          n89 = Unbundle By Name(w648) -> ("Step motor ID"=w623:string, "SMname"=w647:string, "Loft"=w646:u16, "wait for input sygnal to start"=w645:bool, "use slow start/stop"=w644:bool, "units name"=w643:string, "Maximum speed"=w642:dbl, "speed"=w641:dbl, "step"=w640:u8, "point 1 ticks"=w639:i32, "point 2 ticks"=w638:i32, "point 1 units"=w637:dbl, "point 2 units"=w636:dbl, "Trailer 1 standoff"=w635:dbl, "Zero Value"=w634:dbl, "Destination Position"=w633:dbl, "force loft"=w632:bool, "power off when stop"=w631:bool, "POff delay"=w630:dbl, "positioner name"=w629:string, "R, Ohm"=w627:dbl, "I, mA"=w626:dbl, "Positioner's Type"=w625:u16, "Reset Direction"=w624:bool, "Manufacturer"=w622:string, "Model"=w621:string, "Scheme"=w620:string)
          n90 = Bundle By Name(cluster=w619, "Step motor ID"=w623, "SMname"=w647, "Backlash"=w646, "wait for input sygnal to start"=w645, "use slow start/stop"=w644, "units name"=w643, "Maximum speed"=w642, "speed"=w641, "step"=w640, "point 1 ticks"=w639, "point 2 ticks"=w638, "point 1 units"=w637, "point 2 units"=w636, "Limit Switch standoff"=w635, "Zero Value"=w634, "Destination Position"=w633, "force backlash"=w632, "power off when stop"=w631, "POff delay"=w630, "positioner name"=w629, "R, Ohm"=w627, "I, mA"=w626, "Positioner's Type"=w625, "Reset Direction"=w624, "Manufacturer"=w622, "Model"=w621, "Scheme"=w620) -> (w628:T5)
        }
      }
    }
    frame "1.23", "1.24", "1.25", "1.26" {
      w666 = T12 {"Delay 1"=3, "Delay 2"=3, "RefINTimeout"=6579, "BTIMEOUT 1"=6579, "BTIMEOUT 2"=13158, "BTIMEOUT 3"=13158, "BTIMEOUT 4"=13158, "BTIMEOUT R"=6579, "BTIMEOUT D"=1974, "Min period"=63536, "BTO1P"=25536, "BTO2P"=55536, "BTO3P"=61536, "BTO4P"=63536, "Max Loft"=1024, "Start Pos"=0, "RTDelta"=12800, "RTMinError"=320, "Maximum temperature"=23832, "sync duration"=5, "LoftPeriod"=25536}  # SetParams Defalut
      w667 = T19 {"buttons off"=FALSE, "RefIin current"=TRUE, "power off and make a whole step"=TRUE, "emergency power off"=FALSE, "trailer 1 true state"=FALSE, "trailer 2 true state"=FALSE, "Rotary Transducer TRUE state"=TRUE, "trailers swap"=TRUE, "trailer 1 operation enabled"=TRUE, "trailer 2 operation enabled"=TRUE, "Rotary Transducer Operation enabled"=FALSE, "Rotary Transducer Operation select"=TRUE, "Button 1 TRUE state"=FALSE, "Button 2 TRUE state"=FALSE, "Buttons are Swapped"=FALSE, "Reset Rotary Transducer Check Positions"=TRUE, "Output Syncronization Enabled"=FALSE, "reset output sync count"=FALSE, "Sync operation true-one time, false - many times"=FALSE, "Sync count"=50, "power state"=TRUE, "Const TTL output"=FALSE}  # SetMode defalults
      n91 = Bundle("SetMode defalults"=w667, "SetParams Defalut"=w666, "Position Default"=T7 {"cur pos units"=0.0, "set cur pos units value"=0.0, "lo limit units"=-33554428.0, "hi limit units"=33554427.78, "cur pos ticks"=0, "set cur pos ticks value"=0, "lo limit ticks"=-2147483648, "hi limit ticks"=2147483647, "Minimal Value"=-2147483648.0, "Maximal Value"=2147483647.0}, "GoToPlus default"=T8 {"Step motor ID"="0000000000000001", "SMname"="XYZ", "Loft"=0, "wait for input sygnal to start"=FALSE, "use slow start/stop"=TRUE, "units name"="steps", "Maximum speed"=5000.0, "speed"=1500.0, "step"=3, "point 1 ticks"=0, "point 2 ticks"=64, "point 1 units"=0.0, "point 2 units"=1.0, "Trailer 1 standoff"=0.0, "Zero Value"=0.0, "Destination Position"=0.0, "force loft"=FALSE, "power off when stop"=FALSE, "POff delay"=600.0, "positioner name"="Linear", "R, Ohm"=0.0, "I, mA"=0.0, "Positioner's Type"=0, "Reset Direction"=FALSE, "Manufacturer"="Unknown", "Model"="Unknown", "Scheme"="4Wire", "FirmwareVer"="unknown"}) -> (w665:T20)  [unwired: 1 in]
      n92 = Unflatten From String(type=w665, binary string=w664) -> (value=w663:T20)  [unwired: 3 in, 2 out]
      n93 = Unbundle(w663) -> ("SetMode defalults"=w662:T19, "SetParams Defalut"=w659:T12, "Position Default"=w658:T7, "GoToPlus default"=w656:T8)
      n94 = stacked-sequence {
        tunnel: w662 -> [w692 _ _ _]
        tunnel: [w670 _ _ _] -> w661
        tunnel: [_ w730 _ _] -> w660
        tunnel: w659 -> [_ w729 _ _]
        tunnel: w658 -> [_ _ w738 _]
        tunnel: [_ _ w737 _] -> w657
        tunnel: w656 -> [_ _ _ w776]
        tunnel: [_ _ _ w756] -> w655
        tunnel: w652 -> [_ _ _ w747]
        tunnel: w651 -> [w668 _ _ _]
        tunnel: w650 -> [_ w728 _ _]
        tunnel: w649 -> [_ _ w734 _]
        frame #0 {
          n95 = Unbundle By Name(w692) -> ("buttons off"=w691:bool, "RefIin current"=w690:bool, "power off and make a whole step"=w689:bool, "emergency power off"=w688:bool, "trailer 1 true state"=w687:bool, "trailer 2 true state"=w686:bool, "Rotary Transducer TRUE state"=w685:bool, "trailers swap"=w684:bool, "trailer 1 operation enabled"=w683:bool, "trailer 2 operation enabled"=w682:bool, "Rotary Transducer Operation enabled"=w681:bool, "Rotary Transducer Operation select"=w680:bool, "Button 1 TRUE state"=w679:bool, "Button 2 TRUE state"=w678:bool, "Buttons are Swapped"=w677:bool, "Reset Rotary Transducer Check Positions"=w676:bool, "Output Syncronization Enabled"=w675:bool, "reset output sync count"=w673:bool, "Sync operation true-one time, false - many times"=w674:bool, "Sync count"=w672:u32, "power state"=w671:bool, "Const TTL output"=w669:bool)
          n96 = Bundle By Name(cluster=w668, "Turn Buttons Off"=w691, "Reduce Current"=w690, "Power Off and Make a Whole Step"=w689, "Emergency Power Off"=w688, "Limit Switch 1 True State"=w687, "Limit Switch 2 True State"=w686, "Rotary Transducer TRUE State"=w685, "Swap Limit Switches"=w684, "Limit Switch 1 Operation Enabled"=w683, "Limit Switch 2 Operation Enabled"=w682, "Rotary Transducer Operation Enabled"=w681, "Rotary Transducer Operation Select"=w680, "Button 1 True State"=w679, "Button 2 True State"=w678, "Swap Buttons"=w677, "Reset Rotary Transducer Check Positions"=w676, "Output Syncronization Enabled"=w675, "Reset Output Sync Count"=w673, "Sync Operation"=w674, "Sync Count"=w672, "Power"=w671, "Invert Sync Polarity"=w669) -> (w670:T4)
        }
        frame #1 {
          n97 = Unbundle By Name(w729) -> ("Delay 1"=w698:u8, "Delay 2"=w700:u8, "RefINTimeout"=w727:u16, "BTIMEOUT 1"=w726:u16, "BTIMEOUT 2"=w725:u16, "BTIMEOUT 3"=w724:u16, "BTIMEOUT 4"=w723:u16, "BTIMEOUT R"=w722:u16, "BTIMEOUT D"=w721:u16, "Min period"=w713:u16, "BTO1P"=w712:u16, "BTO2P"=w711:u16, "BTO3P"=w710:u16, "BTO4P"=w709:u16, "Max Loft"=w733:u16, "Start Pos"=w732:i32, "RTDelta"=w696:u16, "RTMinError"=w695:u16, "Maximum temperature"=w701:u16, "sync duration"=w731:u8, "LoftPeriod"=w708:u16)
          n98 = call "Calibrate Ticks 2 Timeouts (uSMC).vi"("Buttons Timeout 1 (ticks)"=w726, "Reduce Current Timeout (ticks)"=w727, "Buttons Timeout 2 (ticks)"=w725, "Buttons Timeout 3 (ticks)"=w724, "Buttons Timeout 4 (ticks)"=w723, "Buttons Timeout Reset (ticks)"=w722, "Buttons Timeout DblClick (ticks)"=w721) -> ("Reduce Current Timeout (ms)"=w720:u16, "Buttons Timeout 1 (ms)"=w719:u16, "Buttons Timeout 2 (ms)"=w718:u16, "Buttons Timeout 3 (ms)"=w717:u16, "Buttons Timeout 4 (ms)"=w716:u16, "Buttons Timeout DblClick (ms)"=w714:u16, "Buttons Timeout Reset (ms)"=w715:u16)  [unwired: 2 in]
          n99 = call "Calibrate Ticks 2 Buttons Speed (uSMC).vi"("Backlash Speed (ticks)"=w708, "Reset Speed (ticks)"=w713, "Buttons Speed 4 (ticks)"=w709, "Buttons Speed 3 (ticks)"=w710, "Buttons Speed 2 (ticks)"=w711, "Buttons Speed 1 (ticks)"=w712) -> ("Buttons Speed 4 (Full Steps/Sec)"=w706:u16, "Buttons Speed 3 (Full Steps/Sec)"=w705:u16, "Buttons Speed 2 (Full Steps/Sec)"=w704:u16, "Buttons Speed 1 (Full Steps/Sec)"=w703:u16, "Backlash Speed (Full Steps/Sec)"=w707:u16, "Reset Speed (Full Steps/Sec)"=w702:u16)
          n100 = call "Calibrate Ticks 2 Acceleration (uSMC).vi"("Acceleration (ticks)"=w700) -> ("Acceleration (ms)"=w699:u16)
          n101 = call "Calibrate Ticks 2 Acceleration (uSMC).vi"("Acceleration (ticks)"=w698) -> ("Acceleration (ms)"=w697:u16)
          n102 = call "Calibrate Ticks 2 RT Parameters (uSMC).vi"("RTMinError (ticks)"=w695, "RTDelta (ticks)"=w696) -> ("RTMinError (a.u.)"=w693:u16, "RTDelta (a.u.)"=w694:u16)
          n103 = Bundle By Name(cluster=w728, "Acceleration Time"=w697, "Deceleration Time"=w699, "Reduce Current Timeout"=w720, "Buttons Timeout 1"=w719, "Buttons Timeout 2"=w718, "Buttons Timeout 3"=w717, "Buttons Timeout 4"=w716, "Buttons Timeout Reset"=w715, "Buttons Timeout DblClick"=w714, "Reset Speed"=w702, "Buttons Speed 1"=w703, "Buttons Speed 2"=w704, "Buttons Speed 3"=w705, "Buttons Speed 4"=w706, "Max Backlash"=w733, "Start Pos"=w732, "RTdelta"=w694, "RTMinError"=w693, "Maximum Temperature"=w701, "Sync Duration"=w731, "Backlash Speed"=w707) -> (w730:T2)
        }
        frame #2 {
          n104 = Unbundle By Name(w738) -> ("cur pos units"=w746:dbl, "set cur pos units value"=w745:dbl, "lo limit units"=w744:dbl, "hi limit units"=w743:dbl, "cur pos ticks"=w742:i32, "set cur pos ticks value"=w741:i32, "lo limit ticks"=w740:i32, "hi limit ticks"=w739:i32, "Minimal Value"=w736:dbl, "Maximal Value"=w735:dbl)
          n105 = Bundle By Name(cluster=w734, "Cur Pos Units"=w746, "Set Cur Pos units"=w745, "Lo Limit Units"=w744, "Hi Limit Units"=w743, "Cur Pos Ticks"=w742, "Set Cur Pos ticks"=w741, "Lo Limit Ticks"=w740, "Hi Limit Ticks"=w739, "Minimal Value"=w736, "Maximal Value"=w735) -> (w737:T3)
        }
        frame #3 {
          n106 = Unbundle By Name(w776) -> ("Step motor ID"=w751:string, "SMname"=w775:string, "Loft"=w774:u16, "wait for input sygnal to start"=w773:bool, "use slow start/stop"=w772:bool, "units name"=w771:string, "Maximum speed"=w770:dbl, "speed"=w769:dbl, "step"=w768:u8, "point 1 ticks"=w767:i32, "point 2 ticks"=w766:i32, "point 1 units"=w765:dbl, "point 2 units"=w764:dbl, "Trailer 1 standoff"=w763:dbl, "Zero Value"=w762:dbl, "Destination Position"=w761:dbl, "force loft"=w760:bool, "power off when stop"=w759:bool, "POff delay"=w758:dbl, "positioner name"=w757:string, "R, Ohm"=w755:dbl, "I, mA"=w754:dbl, "Positioner's Type"=w753:u16, "Reset Direction"=w752:bool, "Manufacturer"=w750:string, "Model"=w749:string, "Scheme"=w748:string)
          n107 = Bundle By Name(cluster=w747, "Step motor ID"=w751, "SMname"=w775, "Backlash"=w774, "wait for input sygnal to start"=w773, "use slow start/stop"=w772, "units name"=w771, "Maximum speed"=w770, "speed"=w769, "step"=w768, "point 1 ticks"=w767, "point 2 ticks"=w766, "point 1 units"=w765, "point 2 units"=w764, "Limit Switch standoff"=w763, "Zero Value"=w762, "Destination Position"=w761, "force backlash"=w760, "power off when stop"=w759, "POff delay"=w758, "positioner name"=w757, "R, Ohm"=w755, "I, mA"=w754, "Positioner's Type"=w753, "Reset Direction"=w752, "Manufacturer"=w750, "Model"=w749, "Scheme"=w748) -> (w756:T5)
        }
      }
    }
    frame "1.27", "1.28", "1.29", "1.30", "1.31", "1.32", "1.33", "1.34" {
      n108 = Bundle("Mode Defalults"=T9 {"Turn Buttons Off"=FALSE, "Reduce Current"=TRUE, "Power Off and Make a Whole Step"=TRUE, "Emergency Power Off"=FALSE, "Trailer 1 True State"=FALSE, "Trailer 2 True State"=FALSE, "Rotary Transducer TRUE State"=TRUE, "Swap Trailers"=TRUE, "Trailer 1 Operation Enabled"=TRUE, "Trailer 2 Operation Enabled"=TRUE, "Rotary Transducer Operation Enabled"=FALSE, "Rotary Transducer Operation Select"=TRUE, "Button 1 True State"=FALSE, "Button 2 True State"=FALSE, "Swap Buttons"=FALSE, "Reset Rotary Transducer Check Positions"=TRUE, "Output Syncronization Enabled"=FALSE, "Reset Output Sync Count"=FALSE, "Sync Operation"=FALSE, "Sync Count"=50, "Power"=TRUE, "Invert Sync Polarity"=FALSE, "Use Encoder"=FALSE, "Invert Encoder Direction"=FALSE, "Reset Encoder To 0"=FALSE, "Reset SM Enc Pos to Enc Pos"=FALSE}, "Parameters Defalut"=T2 {"Acceleration Time"=38, "Deceleration Time"=38, "Reduce Current Timeout"=1000, "Buttons Timeout 1"=500, "Buttons Timeout 2"=1000, "Buttons Timeout 3"=1500, "Buttons Timeout 4"=2000, "Buttons Timeout Reset"=2000, "Buttons Timeout DblClick"=294, "Reset Speed"=64, "Buttons Speed 1"=3, "Buttons Speed 2"=13, "Buttons Speed 3"=32, "Buttons Speed 4"=64, "Max Backlash"=1024, "Start Pos"=0, "RTdelta"=200, "RTMinError"=5, "Maximum Temperature"=70, "Sync Duration"=5, "Backlash Speed"=3, "EncVSCP"=10, "Steps Per Revolution"=0, "Encoder Pulses Per Rev-on"=0}, "Position Default"=T7 {"cur pos units"=0.0, "set cur pos units value"=0.0, "lo limit units"=-33554428.0, "hi limit units"=33554427.78, "cur pos ticks"=0, "set cur pos ticks value"=0, "lo limit ticks"=-2147483648, "hi limit ticks"=2147483647, "Minimal Value"=-2147483648.0, "Maximal Value"=2147483647.0}, "GoToPlus default"=T8 {"Step motor ID"="0000000000000001", "SMname"="XYZ", "Loft"=0, "wait for input sygnal to start"=FALSE, "use slow start/stop"=TRUE, "units name"="steps", "Maximum speed"=5000.0, "speed"=1500.0, "step"=3, "point 1 ticks"=0, "point 2 ticks"=64, "point 1 units"=0.0, "point 2 units"=1.0, "Trailer 1 standoff"=0.0, "Zero Value"=0.0, "Destination Position"=0.0, "force loft"=FALSE, "power off when stop"=FALSE, "POff delay"=600.0, "positioner name"="Linear", "R, Ohm"=0.0, "I, mA"=0.0, "Positioner's Type"=0, "Reset Direction"=FALSE, "Manufacturer"="Unknown", "Model"="Unknown", "Scheme"="4Wire", "FirmwareVer"="unknown"}) -> (w796:T21)  [unwired: 1 in]
      n109 = Unflatten From String(type=w796, binary string=w795) -> (value=w794:T21, error out=w777:errorcluster)  [unwired: 3 in, 1 out]
      n110 = Unbundle(w794) -> ("Mode Defalults"=w793:T9, "Parameters Defalut"=w790:T2, "Position Default"=w789:T7, "GoToPlus default"=w787:T8)
      n111 = stacked-sequence {
        tunnel: w793 -> [w825 _ _ _]
        tunnel: [w803 _ _ _] -> w792
        tunnel: [_ w866 _ _] -> w791
        tunnel: w790 -> [_ w865 _ _]
        tunnel: w789 -> [_ _ w874 _]
        tunnel: [_ _ w873 _] -> w788
        tunnel: w787 -> [_ _ _ w912]
        tunnel: [_ _ _ w892] -> w786
        tunnel: w783 -> [_ _ _ w883]
        tunnel: w782 -> [w801 _ _ _]
        tunnel: w781 -> [_ w864 _ _]
        tunnel: w780 -> [_ _ w870 _]
        frame #0 {
          n112 = Unbundle By Name(w825) -> ("Turn Buttons Off"=w824:bool, "Reduce Current"=w823:bool, "Power Off and Make a Whole Step"=w822:bool, "Emergency Power Off"=w821:bool, "Trailer 1 True State"=w820:bool, "Trailer 2 True State"=w819:bool, "Rotary Transducer TRUE State"=w818:bool, "Swap Trailers"=w817:bool, "Trailer 1 Operation Enabled"=w816:bool, "Trailer 2 Operation Enabled"=w815:bool, "Rotary Transducer Operation Enabled"=w814:bool, "Rotary Transducer Operation Select"=w813:bool, "Button 1 True State"=w812:bool, "Button 2 True State"=w811:bool, "Swap Buttons"=w810:bool, "Reset Rotary Transducer Check Positions"=w809:bool, "Output Syncronization Enabled"=w808:bool, "Reset Output Sync Count"=w806:bool, "Sync Operation"=w807:bool, "Sync Count"=w805:u32, "Power"=w804:bool, "Invert Sync Polarity"=w802:bool, "Use Encoder"=w800:bool, "Invert Encoder Direction"=w799:bool, "Reset Encoder To 0"=w798:bool, "Reset SM Enc Pos to Enc Pos"=w797:bool)
          n113 = Bundle By Name(cluster=w801, "Turn Buttons Off"=w824, "Reduce Current"=w823, "Power Off and Make a Whole Step"=w822, "Emergency Power Off"=w821, "Limit Switch 1 True State"=w820, "Limit Switch 2 True State"=w819, "Rotary Transducer TRUE State"=w818, "Swap Limit Switches"=w817, "Limit Switch 1 Operation Enabled"=w816, "Limit Switch 2 Operation Enabled"=w815, "Rotary Transducer Operation Enabled"=w814, "Rotary Transducer Operation Select"=w813, "Button 1 True State"=w812, "Button 2 True State"=w811, "Swap Buttons"=w810, "Reset Rotary Transducer Check Positions"=w809, "Output Syncronization Enabled"=w808, "Reset Output Sync Count"=w806, "Sync Operation"=w807, "Sync Count"=w805, "Power"=w804, "Invert Sync Polarity"=w802, "Use Encoder"=w800, "Invert Encoder Direction"=w799, "Reset Encoder To 0"=w798, "Reset SM Enc Pos to Enc Pos"=w797) -> (w803:T4)
        }
        frame #1 {
          n114 = Unbundle By Name(w865) -> ("Acceleration Time"=w835:u8, "Deceleration Time"=w837:u8, "Reduce Current Timeout"=w863:u16, "Buttons Timeout 1"=w862:u16, "Buttons Timeout 2"=w861:u16, "Buttons Timeout 3"=w860:u16, "Buttons Timeout 4"=w859:u16, "Buttons Timeout Reset"=w858:u16, "Buttons Timeout DblClick"=w857:u16, "Reset Speed"=w849:u16, "Buttons Speed 1"=w848:u16, "Buttons Speed 2"=w847:u16, "Buttons Speed 3"=w846:u16, "Buttons Speed 4"=w845:u16, "Max Backlash"=w869:u16, "Start Pos"=w868:i32, "RTdelta"=w833:u16, "RTMinError"=w832:u16, "Maximum Temperature"=w826:u16, "Sync Duration"=w867:u8, "Backlash Speed"=w844:u16, "EncVSCP"=w829:u8, "Steps Per Revolution"=w828:i32, "Encoder Pulses Per Rev-on"=w827:i32)
          n115 = call "Calibrate Ticks 2 Timeouts (uSMC).vi"("Buttons Timeout 1 (ticks)"=w862, "Reduce Current Timeout (ticks)"=w863, "Buttons Timeout 2 (ticks)"=w861, "Buttons Timeout 3 (ticks)"=w860, "Buttons Timeout 4 (ticks)"=w859, "Buttons Timeout Reset (ticks)"=w858, "Buttons Timeout DblClick (ticks)"=w857) -> ("Reduce Current Timeout (ms)"=w856:u16, "Buttons Timeout 1 (ms)"=w855:u16, "Buttons Timeout 2 (ms)"=w854:u16, "Buttons Timeout 3 (ms)"=w853:u16, "Buttons Timeout 4 (ms)"=w852:u16, "Buttons Timeout DblClick (ms)"=w850:u16, "Buttons Timeout Reset (ms)"=w851:u16)  [unwired: 2 in]
          n116 = call "Calibrate Ticks 2 Buttons Speed (uSMC).vi"("Backlash Speed (ticks)"=w844, "Reset Speed (ticks)"=w849, "Buttons Speed 4 (ticks)"=w845, "Buttons Speed 3 (ticks)"=w846, "Buttons Speed 2 (ticks)"=w847, "Buttons Speed 1 (ticks)"=w848) -> ("Buttons Speed 4 (Full Steps/Sec)"=w842:u16, "Buttons Speed 3 (Full Steps/Sec)"=w841:u16, "Buttons Speed 2 (Full Steps/Sec)"=w840:u16, "Buttons Speed 1 (Full Steps/Sec)"=w839:u16, "Backlash Speed (Full Steps/Sec)"=w843:u16, "Reset Speed (Full Steps/Sec)"=w838:u16)
          n117 = call "Calibrate Ticks 2 Acceleration (uSMC).vi"("Acceleration (ticks)"=w837) -> ("Acceleration (ms)"=w836:u16)
          n118 = call "Calibrate Ticks 2 Acceleration (uSMC).vi"("Acceleration (ticks)"=w835) -> ("Acceleration (ms)"=w834:u16)
          n119 = call "Calibrate Ticks 2 RT Parameters (uSMC).vi"("RTMinError (ticks)"=w832, "RTDelta (ticks)"=w833) -> ("RTMinError (a.u.)"=w830:u16, "RTDelta (a.u.)"=w831:u16)
          n120 = Bundle By Name(cluster=w864, "Acceleration Time"=w834, "Deceleration Time"=w836, "Reduce Current Timeout"=w856, "Buttons Timeout 1"=w855, "Buttons Timeout 2"=w854, "Buttons Timeout 3"=w853, "Buttons Timeout 4"=w852, "Buttons Timeout Reset"=w851, "Buttons Timeout DblClick"=w850, "Reset Speed"=w838, "Buttons Speed 1"=w839, "Buttons Speed 2"=w840, "Buttons Speed 3"=w841, "Buttons Speed 4"=w842, "Max Backlash"=w869, "Start Pos"=w868, "RTdelta"=w831, "RTMinError"=w830, "Maximum Temperature"=w826, "Sync Duration"=w867, "Backlash Speed"=w843, "EncVSCP"=w829, "Steps Per Revolution"=w828, "Encoder Pulses Per Rev-on"=w827) -> (w866:T2)
        }
        frame #2 {
          n121 = Unbundle By Name(w874) -> ("cur pos units"=w882:dbl, "set cur pos units value"=w881:dbl, "lo limit units"=w880:dbl, "hi limit units"=w879:dbl, "cur pos ticks"=w878:i32, "set cur pos ticks value"=w877:i32, "lo limit ticks"=w876:i32, "hi limit ticks"=w875:i32, "Minimal Value"=w872:dbl, "Maximal Value"=w871:dbl)
          n122 = Bundle By Name(cluster=w870, "Cur Pos Units"=w882, "Set Cur Pos units"=w881, "Lo Limit Units"=w880, "Hi Limit Units"=w879, "Cur Pos Ticks"=w878, "Set Cur Pos ticks"=w877, "Lo Limit Ticks"=w876, "Hi Limit Ticks"=w875, "Minimal Value"=w872, "Maximal Value"=w871) -> (w873:T3)
        }
        frame #3 {
          n123 = Unbundle By Name(w912) -> ("Step motor ID"=w887:string, "SMname"=w911:string, "Loft"=w910:u16, "wait for input sygnal to start"=w909:bool, "use slow start/stop"=w908:bool, "units name"=w907:string, "Maximum speed"=w906:dbl, "speed"=w905:dbl, "step"=w904:u8, "point 1 ticks"=w903:i32, "point 2 ticks"=w902:i32, "point 1 units"=w901:dbl, "point 2 units"=w900:dbl, "Trailer 1 standoff"=w899:dbl, "Zero Value"=w898:dbl, "Destination Position"=w897:dbl, "force loft"=w896:bool, "power off when stop"=w895:bool, "POff delay"=w894:dbl, "positioner name"=w893:string, "R, Ohm"=w891:dbl, "I, mA"=w890:dbl, "Positioner's Type"=w889:u16, "Reset Direction"=w888:bool, "Manufacturer"=w886:string, "Model"=w885:string, "Scheme"=w884:string)
          n124 = Bundle By Name(cluster=w883, "Step motor ID"=w887, "SMname"=w911, "Backlash"=w910, "wait for input sygnal to start"=w909, "use slow start/stop"=w908, "units name"=w907, "Maximum speed"=w906, "speed"=w905, "step"=w904, "point 1 ticks"=w903, "point 2 ticks"=w902, "point 1 units"=w901, "point 2 units"=w900, "Limit Switch standoff"=w899, "Zero Value"=w898, "Destination Position"=w897, "force backlash"=w896, "power off when stop"=w895, "POff delay"=w894, "positioner name"=w893, "R, Ohm"=w891, "I, mA"=w890, "Positioner's Type"=w889, "Reset Direction"=w888, "Manufacturer"=w886, "Model"=w885, "Scheme"=w884) -> (w892:T5)
        }
      }
    }
    frame "False", Default {
      n125 = Bundle("Mode Defalults"=w917, "Parameters Defalut"=w916, "Position Default"=w915, "StartPlus Default"=w914) -> (w925:T22)  [unwired: 1 in]
      n126 = Unflatten From String(type=w925, binary string=w924) -> (value=w923:T22, error out=w913:errorcluster)  [unwired: 3 in, 1 out]
      n127 = Unbundle(w913) -> ("status"=w918:bool)  [unwired: 2 out]
      n128 = case shown="True" w918 {
        tunnel: w923 -> [w930 _]
        tunnel: [w929 w934] -> w922
        tunnel: [w928 w933] -> w921
        tunnel: [w927 w932] -> w920
        tunnel: [w926 w931] -> w919
        tunnel: w917 -> [_ w934]
        tunnel: w916 -> [_ w933]
        tunnel: w915 -> [_ w932]
        tunnel: w914 -> [_ w931]
        frame False {
          n129 = Unbundle(w930) -> ("Mode Defalults"=w929:T4, "Parameters Defalut"=w928:T2, "Position Default"=w927:T3, "StartPlus Default"=w926:T5)
        }
        frame True {
        }
      }
    }
  }
  n130 = global read "class_data.vi" "Mode Array"() -> (w26:T4[])
  n131 = Array Size(array=w26) -> (size(s)=w25:i32)
  n132 = global read "class_data.vi" "StartPlus Array"() -> (w11:T5[])
  n133 = Decrement(x=w25) -> (x-1=w24:i32)
  n134 = global read "class_data.vi" "Parameters Array"() -> (w31:T2[])
  n135 = global read "class_data.vi" "Position Array"() -> (w30:T23)
  n136 = global read "class_data.vi" "Current State"() -> (w22:T1[])
  n137 = Less Or Equal?(x="SMindex", y=w24) -> ()  [unwired: 1 out]
  n138 = Index Array(array=w11, index="SMindex") -> (element=w10:T5)
  n139 = case shown="True" "replace(false)/insert(true)" {
    tunnel: [w950 w966] -> w14
    tunnel: w31 -> [w949 w965]
    tunnel: [w948 w964] -> w6
    tunnel: w30 -> [w947 w963]
    tunnel: [w946 w962] -> w12
    tunnel: w11 -> [w945 w961]
    tunnel: [w944 w960] -> w18
    tunnel: "SMindex" -> [w937 w952]
    tunnel: w29 -> [w943 w959]
    tunnel: w17 -> [w942 w958]
    tunnel: w28 -> [w941 w957]
    tunnel: w27 -> [w940 w956]
    tunnel: w26 -> [w939 w955]
    tunnel: w22 -> [w938 w954]
    tunnel: [w936 w953] -> w13
    tunnel: T1 {"Current Posistion"=0.0, "CW/CCW"=FALSE, "Speed"=0, "Temperature"=0.0, "Power"=0, "Limit Switch 1"=FALSE, "Limit Switch 2"=FALSE, "After Reset"=FALSE, "Step"=0, "Backlash"=FALSE, "RT Error"=FALSE, "RT State"=FALSE, "Sync In"=FALSE, "Sync Out"=FALSE, "Ext Disconnect"=FALSE, "Usb Powered"=FALSE, "Voltage"=0.0, "Working"=FALSE, "SM Position in Encoder Units"=0, "Encoder Current Position"=0} ("State cluster") -> [w935 w951]
    frame True {
      n140 = Insert Into Array(array=w939, index=w937, new element=w943) -> (w950:T4[])
      n141 = Insert Into Array(array=w949, index=w937, new element=w942) -> (w948:T2[])
      n142 = Insert Into Array(array=w947, index=w937, new element=w941) -> (w946:T23)
      n143 = Insert Into Array(array=w945, index=w937, new element=w940) -> (w944:T5[])
      n144 = Insert Into Array(array=w938, index=w937, new element=w935) -> (w936:T1[])
    }
    frame False {
      n145 = Replace Array Subset(array=w954, new element=w951, index=w952) -> (w953:T1[])
      n146 = Replace Array Subset(array=w955, new element=w959, index=w952) -> (w966:T4[])
      n147 = Replace Array Subset(array=w965, new element=w958, index=w952) -> (w964:T2[])
      n148 = Replace Array Subset(array=w963, new element=w957, index=w952) -> (w962:T23)
      n149 = Replace Array Subset(array=w961, new element=w956, index=w952) -> (w960:T5[])
    }
  }
  n150 = Unbundle By Name(w10) -> ("FirmwareVer"=w9:string, "Step motor ID"=w7:string)
  n151 = Index Array(array=w18, index="SMindex") -> (element=w20:T5)
  n152 = Unbundle By Name(w17) -> ("Maximum Temperature"=w16:u16)
  n153 = Bundle By Name(cluster=w20, "FirmwareVer"=w9, "Step motor ID"=w7) -> (w19:T5)
  n154 = Replace Array Subset(array=w18, new element=w19, index="SMindex") -> (w15:T5[])
  n155 = stacked-sequence {
    tunnel: w16 -> [_ w975]
    tunnel: "SMindex" -> [_ w973]
    tunnel: w15 -> [w970 _]
    tunnel: w14 -> [w969 _]
    tunnel: w13 -> [w968 _]
    tunnel: w12 -> [w967 _]
    tunnel: w6 -> [_ w972]
    frame #0 {
      n156 = global write "class_data.vi" "Mode Array"(w969) -> ()
      n157 = global write "class_data.vi" "StartPlus Array"(w970) -> ()
      n158 = global write "class_data.vi" "Position Array"(w967) -> ()
      n159 = global write "class_data.vi" "Current State"(w968) -> ()
    }
    frame #1 {
      w976 = 70.0 ("y")
      n160 = call "Calibrate Ticks 2 Temperature (uSMC).vi"("SMindex"=w973, "temperature (ticks)"=w975) -> ("Temperature (Cels)"=w974:dbl)
      n161 = Less?(x=w974, y=w976) -> (x < y?=w977:bool)
      n162 = case shown="True" w977 {
        tunnel: w976 -> [_ w981]
        tunnel: w973 -> [_ w982]
        tunnel: w972 -> [w978 w980]
        tunnel: [w978 w979] -> w971
        frame False {
        }
        frame True {
          n163 = Index Array(array=w980, index=w982) -> (element=w983:T2)
          n164 = Bundle By Name(cluster=w983, "Maximum Temperature"=w981) -> (w984:T2)
          n165 = Replace Array Subset(array=w980, new element=w984, index=w982) -> (w979:T2[])
        }
      }
      n166 = global write "class_data.vi" "Parameters Array"(w971) -> ()
    }
  }
